vi "PhotogatePiezoMirror.vi"() -> ()   [LabVIEW 2011]
uses:
  <userlib>/atmcd32d.llb/HSSpeed_type typedef.ctl
  <userlib>/atmcd32d.llb/OutputAmplifier_type typedef.ctl
  <vilib>/vision/Image Controls.llb/IMAQ Image.ctl
  <userlib>/atmcd32d.llb/EMGainMode_mode typedef.ctl
  <userlib>/atmcd32d.llb/Shutter_type typedef.ctl
  <userlib>/atmcd32d.llb/Shutter_mode typedef.ctl
  <vilib>/DAQmx/write.llb/DAQmx Write (Analog 1D DBL NChan 1Samp).vi
  <vilib>/DAQmx/write.llb/DAQmx Write (Analog 2D DBL NChan NSamp).vi
  <vilib>/DAQmx/write.llb/DAQmx Write (Digital Bool 1Line 1Point).vi
  <vilib>/DAQmx/create/channels.llb/DAQmx Create Channel (DO-Digital Output).vi
  <vilib>/DAQmx/create/channels.llb/DAQmx Create Channel (AO-Voltage-Basic).vi
  <vilib>/DAQmx/miscellaneous.llb/DAQmx Fill In Error Info.vi
  <vilib>/DAQmx/configure/timing.llb/DAQmx Timing (Sample Clock).vi
  <vilib>/Utility/inputDevices.llb/closeKeyboard.vi
  <vilib>/Utility/inputDevices.llb/keyboardAcquire.vi
  <vilib>/vision/NI_Vision_Development_Module.lvlib
  MCL libraries/MicroDrive.dll
panel:
  in  "Pattern Tab":enum32{"Page 1"}(tab)
  in  "Reset Pattern":bool
  in  "Camera Tab":T1(tab)
  in  "Shutter control":bool=TRUE
  in  "Run pattern":bool
  in  "Control type":T2(ring)
  in  "Mirror pattern params":T3={"Start radius (V)"=1.0, "End radius (V)"=3.0, "Mirror loop rate (Hz)"=200.0, "Ring duration (s)"=1.0, "Ring center X (V)"=0.0, "Ring center Y(V)"=0.0, "Number of spirals"=3, "Time between \ngates (ms)"=0} {"End radius (V)" format="%0.2f"; "Ring center Y(V)" format="%0.2f"; "Ring center X (V)" format="%0.2f"; "Ring duration (s)" format="%0.2f"; "Mirror loop rate (Hz)" format="%0.2f"; "Start radius (V)" format="%0.2f"}
  out "Piezo mirror position":cluster{dbl[], dbl[]}(graph)
  in  "x10":bool
  in  "/10":bool
  in  "Step Size (um)":dbl
  in  "Left":bool
  in  "Right":bool
  in  "Down":bool
  in  "Up":bool
  in  "Zero lower value":bool
  in  "increase jump step size":bool
  in  "decrease jump step size":bool
  in  "Manual Control":bool=TRUE
  in  "Jump step\nsize (um)":dbl=7.0
  in  "Load ROIs":bool
  in  "Standard Pixel Size":bool=TRUE
  out "Main loop running":dbl
  out "Camera starting":dbl
  in  "ROI 128x128":bool
  in  "Reset Scale":bool
  in  "Kill":bool
  out "buffer size":u32 caption="Buf Size"
  in  "Save Note":bool
  in  ".note text control":string
  out "Temp 2":i32 caption="Temp"
  in  "Previous":bool
  in  "Vend":i32=512
  in  "Vstart":i32=1
  in  "Hend":i32=512
  in  "Hstart":i32=1
  in  "Rotate":bool
  in  "Save":bool
  in  "ROI 512x512":bool
  in  "Live":bool
  out "Rate/Hz":u32
  out "# Saved Fr":i32
  out "Act Rate":sgl caption="Calc/Hz"
  out "# images\nin buffer":u32 caption="Buffer / Load"
  out "Buffer":bool
  in  "Auto Scale":bool
  in  "Slide":cluster{dbl, dbl}(slide)={0.0, 5.408163265306123} scale=461.0..773.0
  out "Image 2":T4(plugin-control)
  in  "Image":bool=TRUE
  out "Updating\nImage":bool
  in  "Start Camera":bool
  in  "Pixel Size (nm)":dbl=107.0 caption="pixel"
  in  "Stop Program":bool
  in  "Close Camera":bool
  in  "Direction to move":dbl(knob)
  in  "Time before pattern starts":u32=2000
  out "Current File":string
  in  "File Name":string="stest"
  in  "Folder":path=path "F:/Vlad/122214"
  in  "Gamepad Option":bool
  in  "Save ROIs":bool
  in  "Move with ROI Line":bool
  in  "Base Multiplication Factor":i32=1
  out "Current Speed Multiplication factor":i32
  in  "Max Speed Multiplication Factor":i32=5
  in  "Velocity (mm/s)":dbl=1.5 format="%.3f"
  in  "base step size (um)":dbl=0.2 format="%.3f"
  out "X-Encoder (mm)":dbl format="%.3f"
  out "Y-Encoder (mm)":dbl format="%.3f"
  in  "Photogate":bool
  in  "Piezo mirror X (V)":dbl(slide)=5.0 scale=0.0..10.0
  in  "Piezo mirror Y (V)":dbl(slide)=5.0 scale=0.0..10.0
  out "Piezo mirror\nloop duration (s)":dbl
  in  "Imaging delay (ms)":sgl
  out "Do Stage Jump":bool
  out "keys pressed":T5(array[ring])
  out "First Key":T6(ring)
  in  "Y Increasing":string(combo)="32"
  in  "Y Decreasing":string(combo)="28"
  in  "X Decreasing":string(combo)="10"
  in  "X Increasing":string(combo)="13"
  out "X Reverse Limit":bool
  out "X Forward Limit":bool
  out "Y Reverse Limit":bool
  out "Y Forward Limit":bool
  in  "Reset Y":bool
  in  "Reset  Both":bool
  in  "Reset X":bool
  in  "Time before stage jump":u32=300
  in  "Convert Files":bool
  in  "Analyze Files":bool
  out "List Analyzed":string[](array[string])
  out "List Not Analyzed":string[](array[string])
  in  "Fan Mode":i32(ring)=2 items=["fan on full", "fan on low", "fan off"]
  out "Actual Expsoure":sgl
  in  "Shutter":u16(ring) items=["Auto", "Open", "Closed"]
  in  "PreAmp":i32(ring)=2 items=["1X", "2.5X", "5.4X"]
  in  "VS Speed":i32(ring)=1 items=["0.3 usec", "0.5 usec", "0.9 usec", "1.7 usec", "3.3 usec"]
  in  "HS Speed":i32(ring)=1 items=["10 MHz", "5 MHz", "3 MHz", "1 MHz"]
  in  "Gain":i32=50
  in  "Exposure(ms)":sgl=100.0 format="%#.2f"
  in  "Temp 3":i32=-80 caption="Temperature"
  out "Camera Closing":bool
  out "Program Closing":bool
  out ".note path":path
  in  "16-bit Display Mapping:Conversion Method":u32(ring)=2 items=["Full Dynamic", "Downshift", "Given Range", "90% Dynamic", "Given Percent Range"]
  out "ref image":T4
  in  "Output Amp":T7
  in  "EMCCD":T8
  out "error out 3":errorcluster
  out "Y #pixels":i32
  out "X #pixels":i32
  out "total #pixels":i32
  in  "Trigger":u32(ring) items=["Internal", "External"]
  out "Camera Initialized":bool
  out "His Hstart":i32=1
  out "His Vstart":i32=1
  out "His Hend":i32=1
  out "His Vend":i32=1
  in  "Keep cooler on":bool
  out "frame rate var":i32
  out "tick var":u32
  out "DLL error code":u32
  out "ref image fake":T4
  out "Temp>0":bool
  in  "Base Path":path=path "F:/Vlad"
  out "Saved ROI":T9
  out "Saving File":bool
  in  "timing source":tag="/Dev1/PFI0"
  # "R      G      B       V"
  # "Notes"
  # "Press Ctrl to create the second ROI"
  # "Camera Settings"
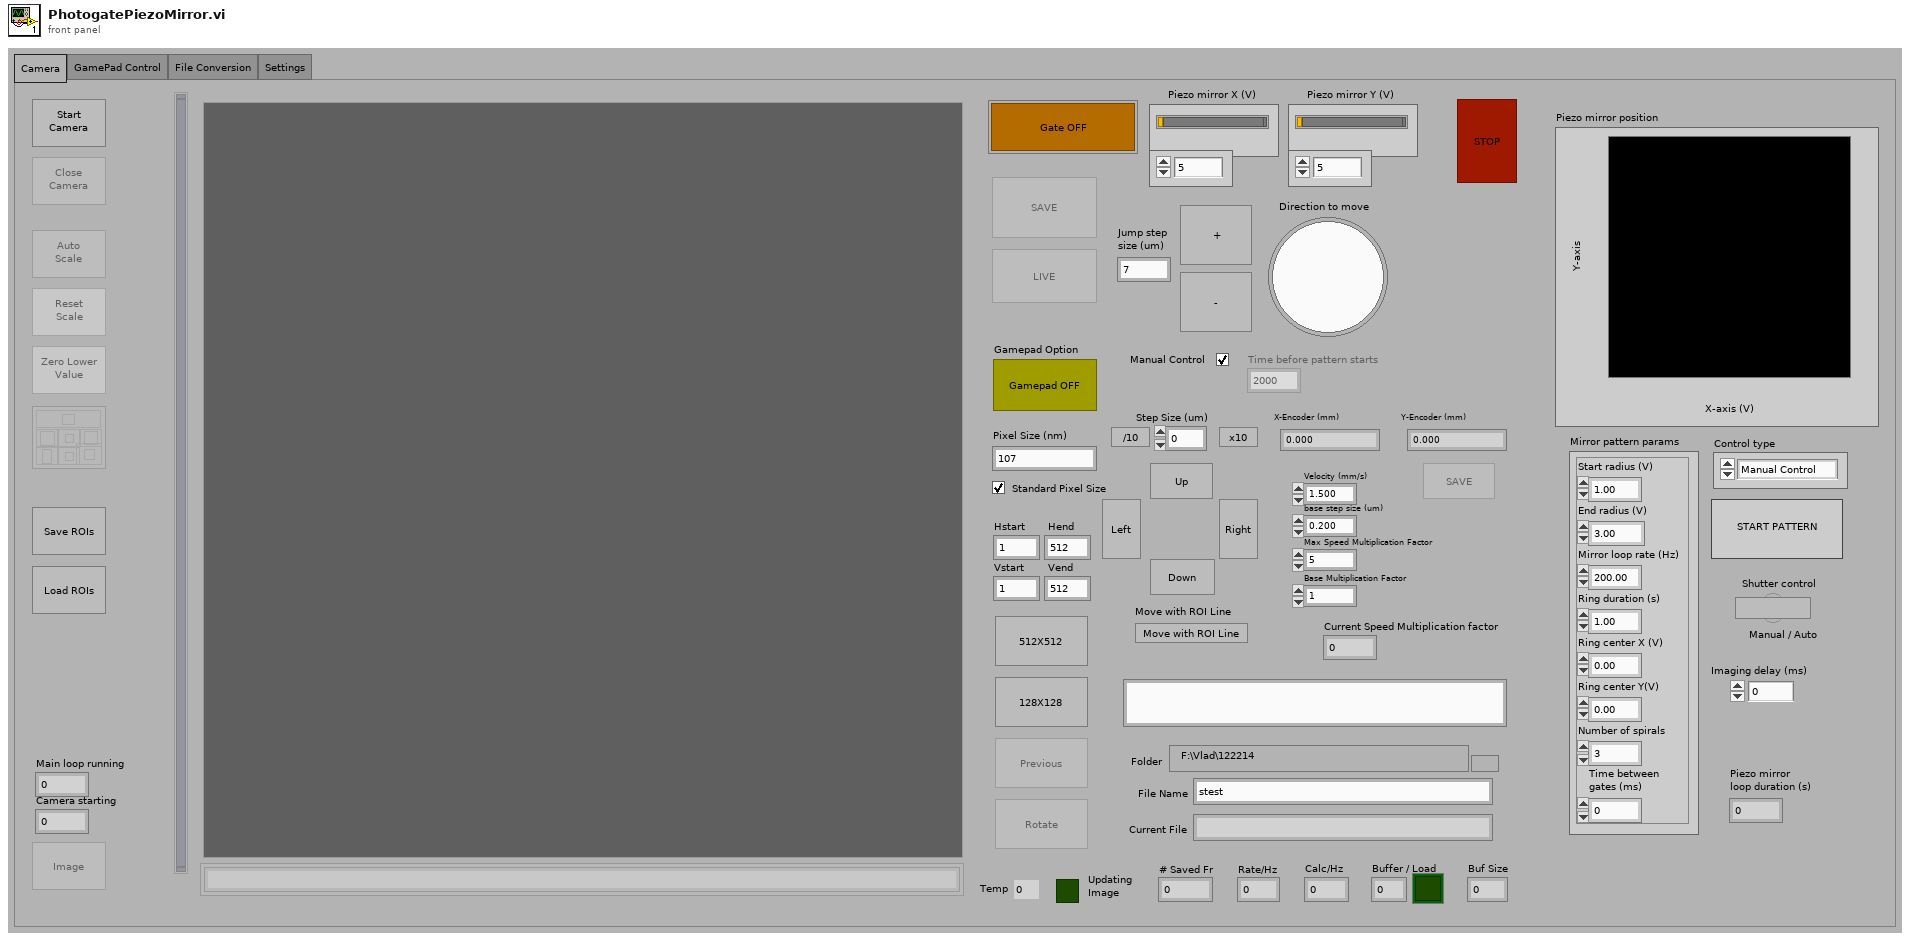
[diagram p1: front panel]
types:
  T1 = enum32{"Camera", "GamePad Control", "File Conversion", "Settings"}
  T2 = enum16{"Manual Control", "Single pattern", "Spiral to circle"}
  T3 = cluster{"Start radius (V)":dbl, "End radius (V)":dbl, "Mirror loop rate (Hz)":dbl, "Ring duration (s)":dbl, "Ring center X (V)":dbl, "Ring center Y(V)":dbl, "Number of spirals":u32, "Time between \ngates (ms)":u32}
  T4 = typedef "IMAQ Image.ctl" = refnum<image>
  T5 = enum16{"0", "1", "2", "3", "4", "5", "6", "7", "8", "9", "A", "B", "C", "D", "E", "F", "G", "H", "I", "J", "K", "L", "M", "N", "O", "P", "Q", "R", "S", "T", "U", "V", "W", "X", "Y", "Z", "F1", "F2", "F3", "F4", "F5", "F6", "F7", "F8", "F9", "F10", "F11", "F12", "F13", "F14", "F15", "ADD", "BACK", "BACKSLASH", "CAPITAL", "COMMA", "DECIMAL", "DELETE", "DIVIDE", "DOWN", "END", "EQUALS", "ESCAPE", "GRAVE (`)", "HOME", "INSERT", "LBRACKET", "LCONTROL", "LEFT", "L ALT", "LSHIFT", "LWIN", "MINUS", "MULTIPLY", "NEXT", "NUMLOCK", "NUMPAD_0", "NUMPAD_1", "NUMPAD_2", "NUMPAD_3", "NUMPAD_4", "NUMPAD_5", "NUMPAD_6", "NUMPAD_7", "NUMPAD_8", "NUMPAD_9", "PAUSE", "PERIOD", "PRIOR (PG UP)", "RBRACKET", "RCONTROL", "RETURN", "RIGHT", "R ALT", "RSHIFT", "RWIN", "SCROLL", "SEMICOLON", "SLASH", "SPACE", "SUBTRACT", "TAB", "UP", "ENTER (num pad)", "' (quote)"}[]
  T6 = enum32{"0", "1", "2", "3", "4", "5", "6", "7", "8", "9", "A", "B", "C", "D", "E", "F", "G", "H", "I", "J", "K", "L", "M", "N", "O", "P", "Q", "R", "S", "T", "U", "V", "W", "X", "Y", "Z", "F1", "F2", "F3", "F4", "F5", "F6", "F7", "F8", "F9", "F10", "F11", "F12", "F13", "F14", "F15", "ADD", "BACK", "BACKSLASH", "CAPITAL", "COMMA", "DECIMAL", "DELETE", "DIVIDE", "DOWN", "END", "EQUALS", "ESCAPE", "GRAVE (`)", "HOME", "INSERT", "LBRACKET", "LCONTROL", "LEFT", "L ALT", "LSHIFT", "LWIN", "MINUS", "MULTIPLY", "NEXT", "NUMLOCK", "NUMPAD_0", "NUMPAD_1", "NUMPAD_2", "NUMPAD_3", "NUMPAD_4", "NUMPAD_5", "NUMPAD_6", "NUMPAD_7", "NUMPAD_8", "NUMPAD_9", "PAUSE", "PERIOD", "PRIOR (PG UP)", "RBRACKET", "RCONTROL", "RETURN", "RIGHT", "R ALT", "RSHIFT", "RWIN", "SCROLL", "SEMICOLON", "SLASH", "SPACE", "SUBTRACT", "TAB", "UP", "ENTER (num pad)", "' (quote)"}
  T7 = typedef "OutputAmplifier_type typedef.ctl" = enum16{"Standard EMCCD gain register", "Conventional CCD register"}
  T8 = typedef "HSSpeed_type typedef.ctl" = enum16{"EM Amp", "Conventional Amp"}
  T9 = cluster{"Global Rectangle":i32[], "Contours":cluster{"Contour Type":u32, "ROI Type":u32, "Points":i32[]}[]}
  T10 = enum8{"Enabled", "Disabled", "Disabled and Grayed Out"}
  T11 = enum16{"open", "replace", "create", "open or create", "replace or create", "replace or create with confirmation"}
  T12 = typedef "Shutter_type typedef.ctl" = enum16{"TTL Low", "TTL High"}
  T13 = typedef "Shutter_mode typedef.ctl" = enum16{"Auto", "Open", "Close"}
  T14 = enum16{"big-endian, network order", "native, host order", "little-endian"}
  T15 = typedef "EMGainMode_mode typedef.ctl" = enum16{"8-bit", "12-bit", "Linear", "Real"}
  T16 = typedef "Image Type" = u32
  T17 = enum16{"0", "1", "2", "3", "4", "5", "6", "7", "8", "9", "A", "B", "C", "D", "E", "F", "G", "H", "I", "J", "K", "L", "M", "N", "O", "P", "Q", "R", "S", "T", "U", "V", "W", "X", "Y", "Z", "F1", "F2", "F3", "F4", "F5", "F6", "F7", "F8", "F9", "F10", "F11", "F12", "F13", "F14", "F15", "ADD", "BACK", "BACKSLASH", "CAPITAL", "COMMA", "DECIMAL", "DELETE", "DIVIDE", "DOWN", "END", "EQUALS", "ESCAPE", "GRAVE (`)", "HOME", "INSERT", "LBRACKET", "LCONTROL", "LEFT", "L ALT", "LSHIFT", "LWIN", "MINUS", "MULTIPLY", "NEXT", "NUMLOCK", "NUMPAD_0", "NUMPAD_1", "NUMPAD_2", "NUMPAD_3", "NUMPAD_4", "NUMPAD_5", "NUMPAD_6", "NUMPAD_7", "NUMPAD_8", "NUMPAD_9", "PAUSE", "PERIOD", "PRIOR (PG UP)", "RBRACKET", "RCONTROL", "RETURN", "RIGHT", "R ALT", "RSHIFT", "RWIN", "SCROLL", "SEMICOLON", "SLASH", "SPACE", "SUBTRACT", "TAB", "UP", "ENTER (num pad)", "' (quote)"}
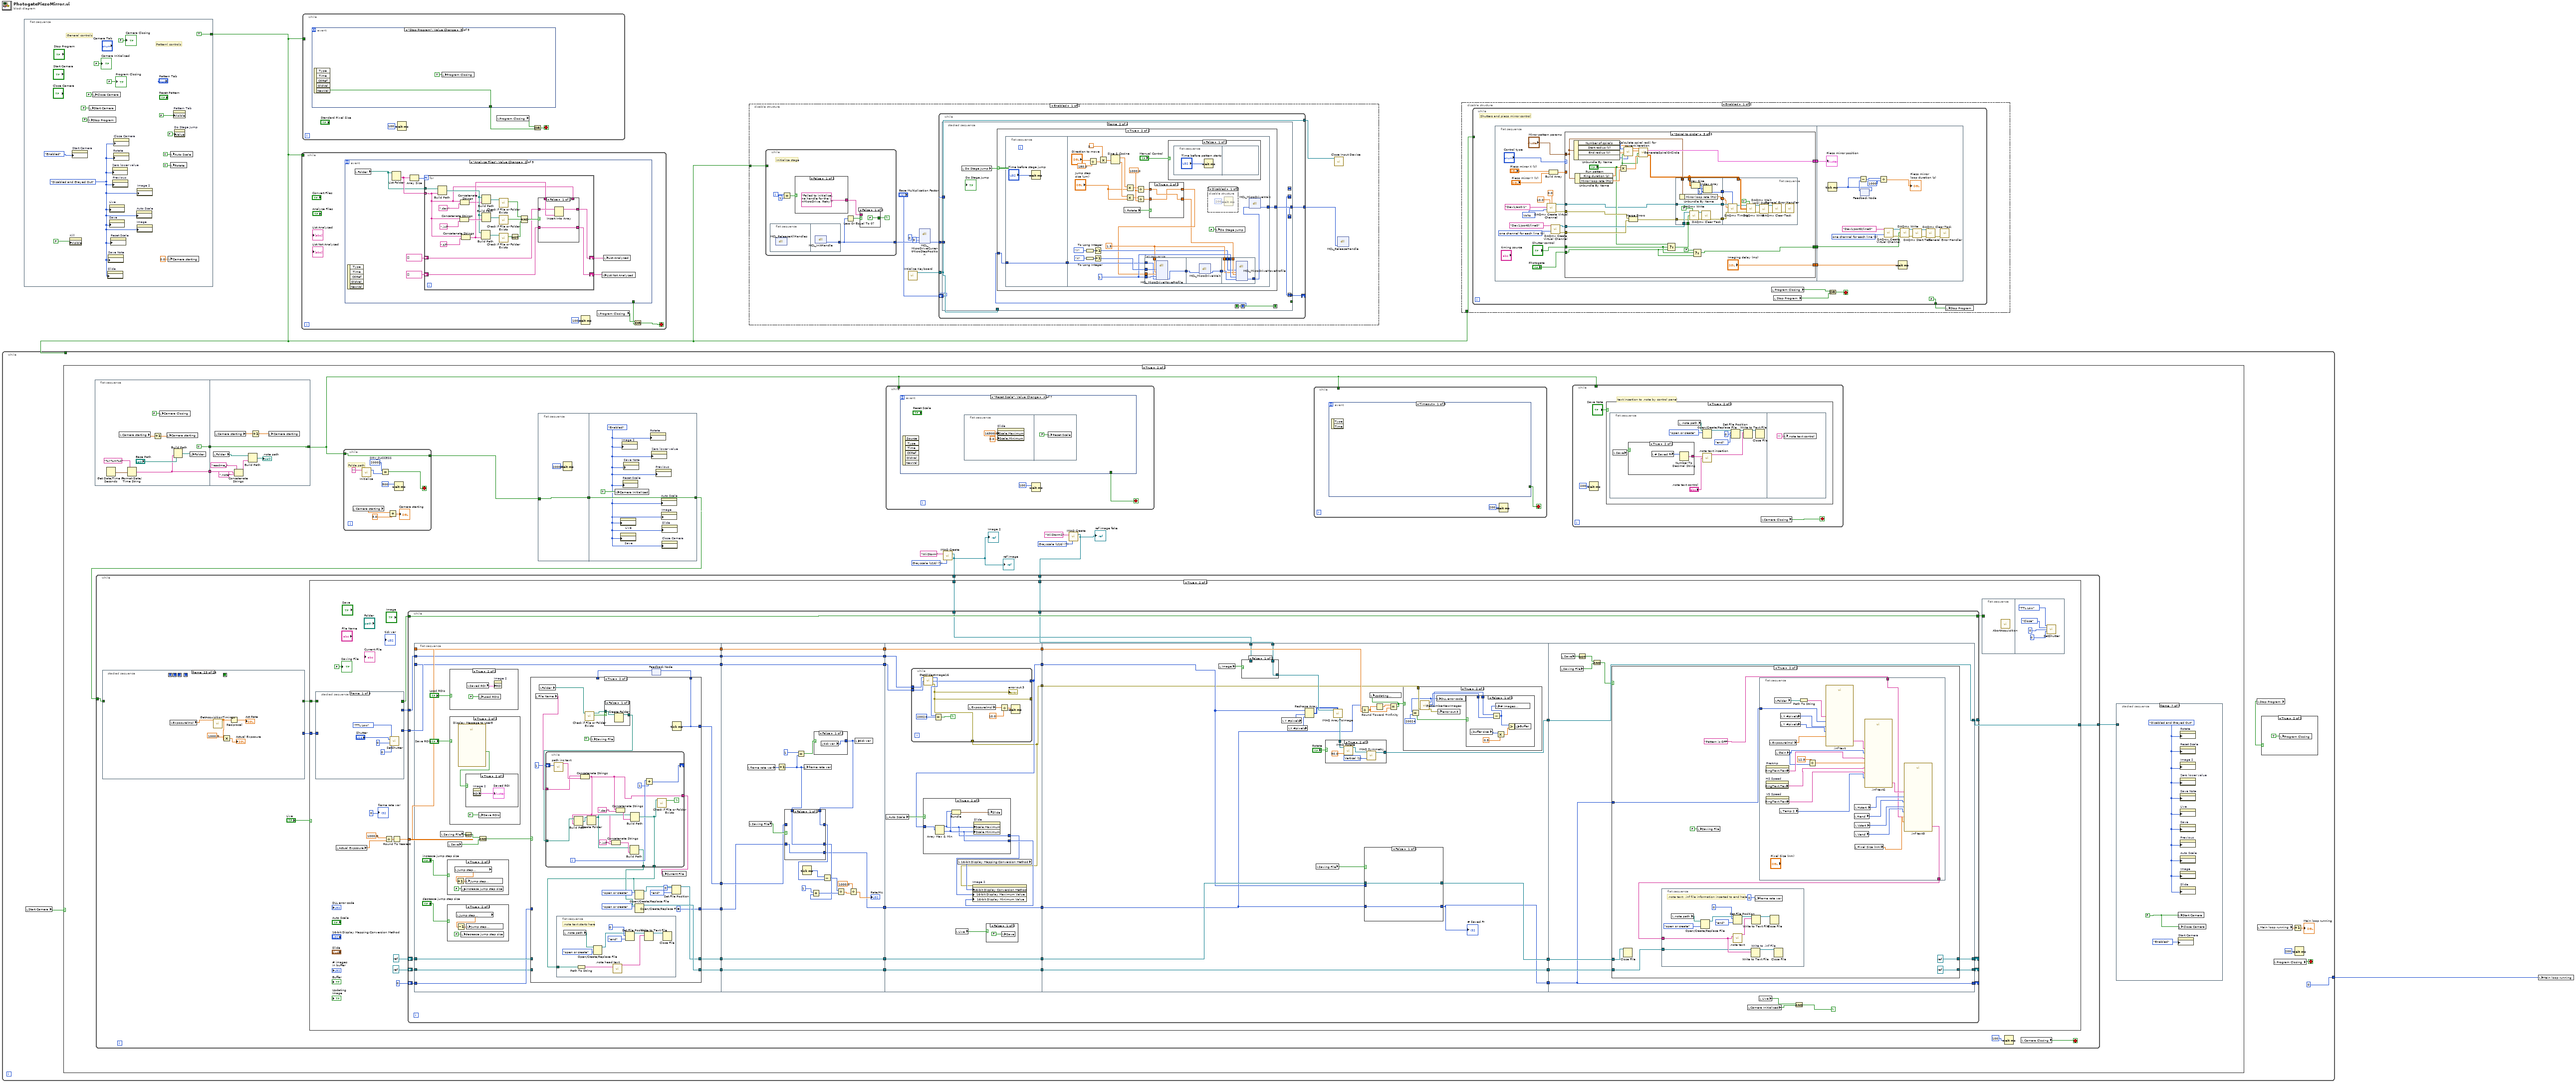
[diagram p0: block diagram]
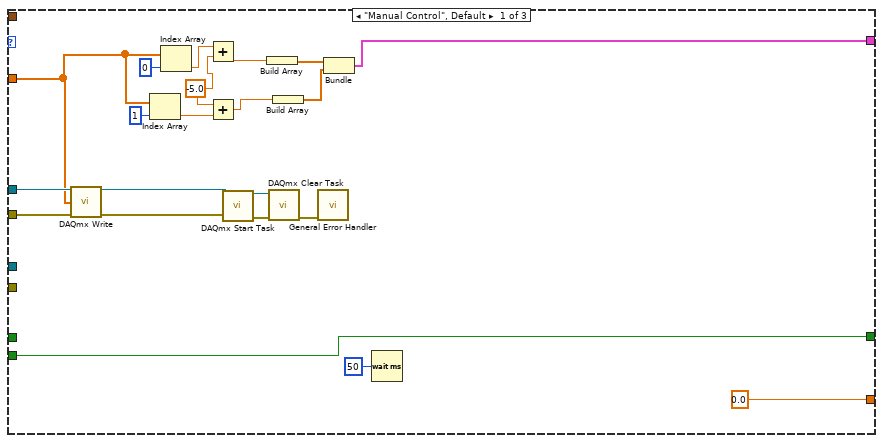
[diagram p2: hidden frame]
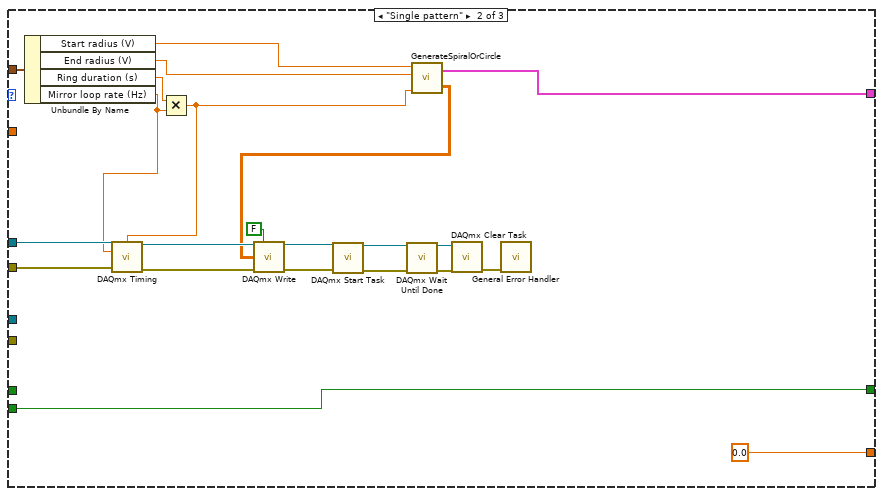
[diagram p3: hidden frame]
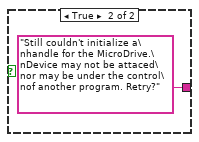
[diagram p5: hidden frame]
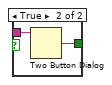
[diagram p6: hidden frame]
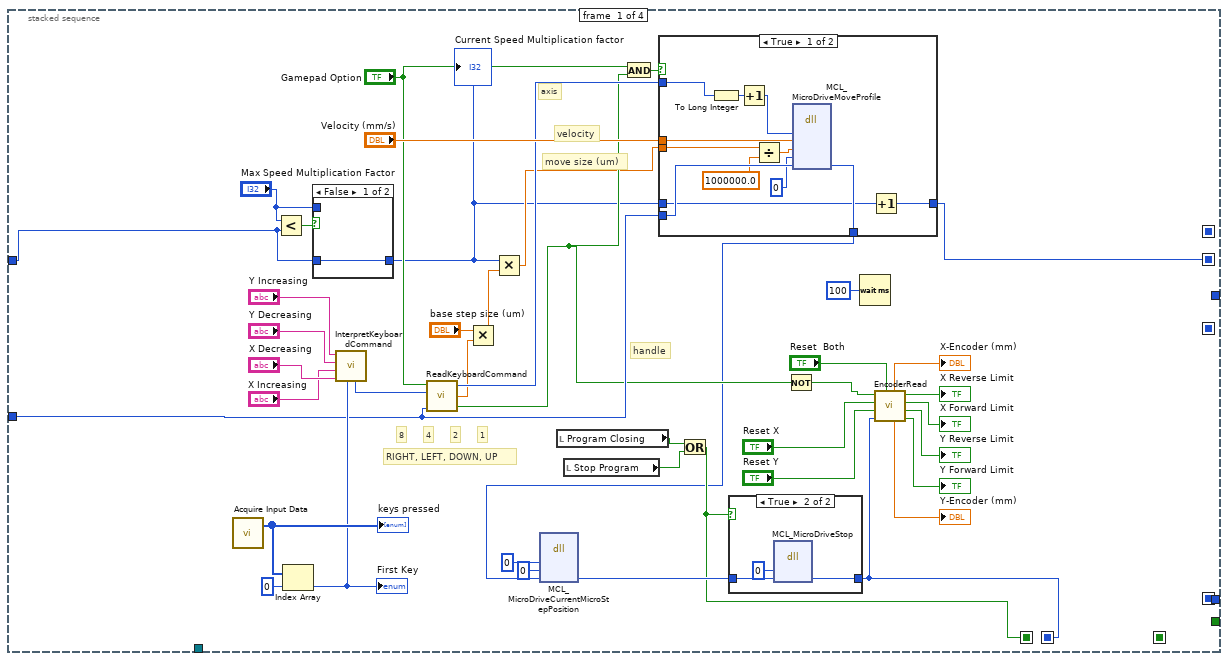
[diagram p7: hidden frame]
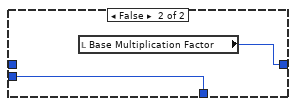
[diagram p9: hidden frame]
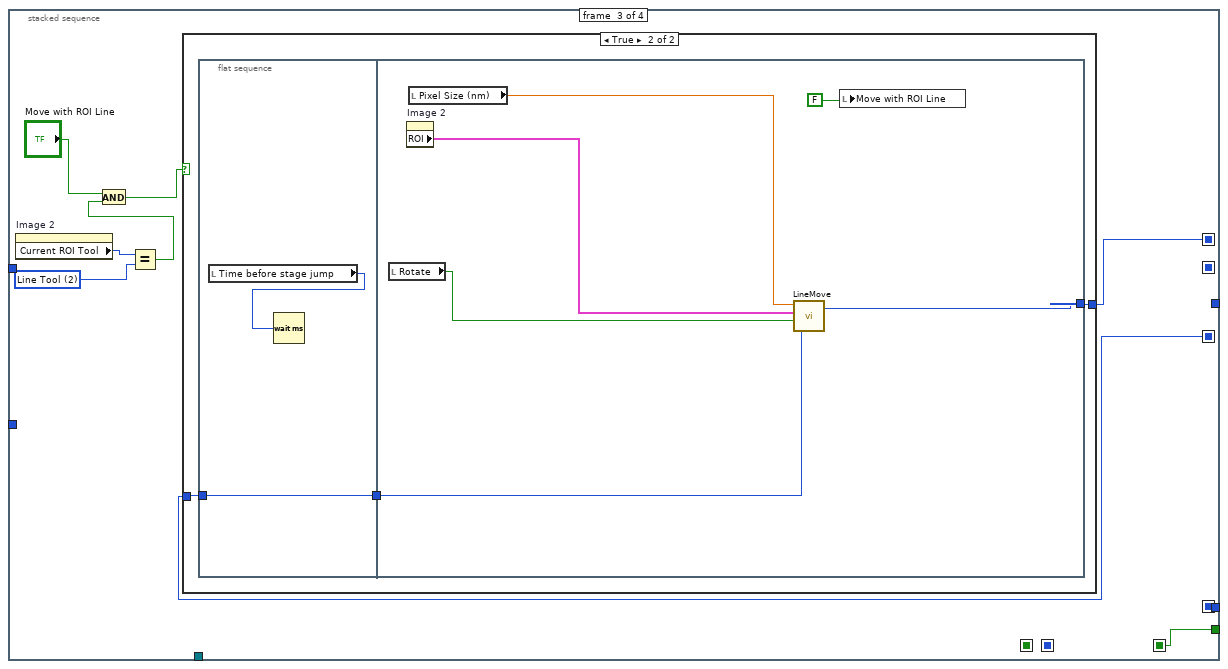
[diagram p15: hidden frame]
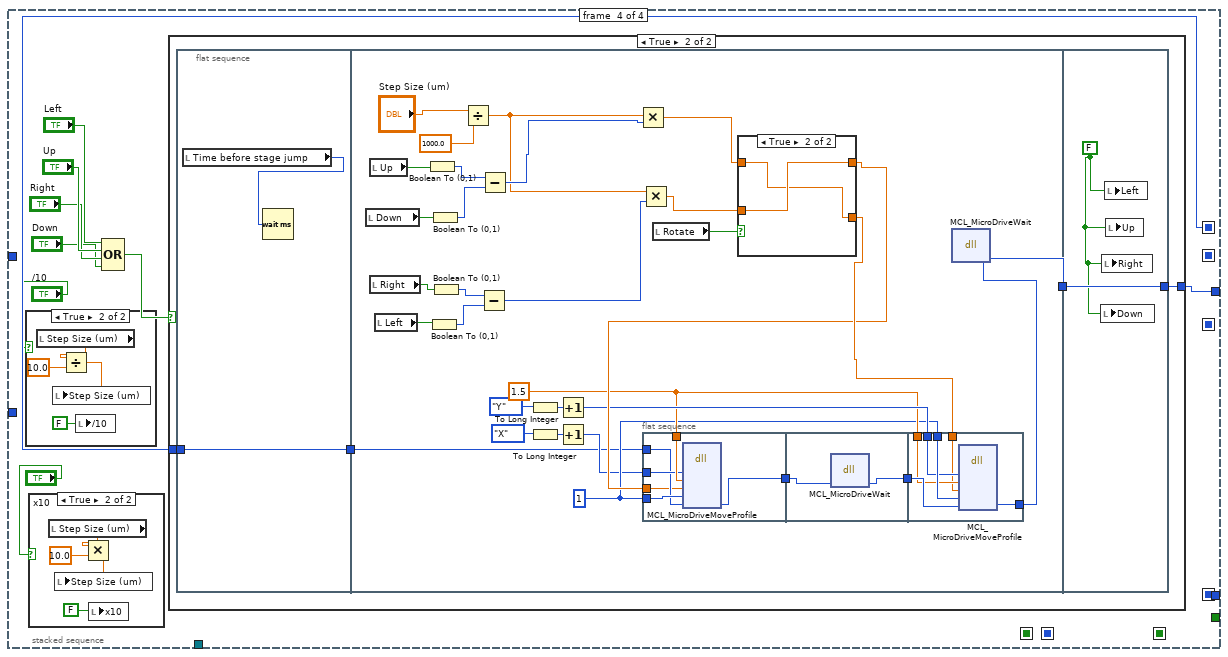
[diagram p17: hidden frame]
diagram:
  n1 = while {
    tunnel: w1 -> [_]
    tunnel: [0] -> w2
    stop <- w7 stop-if-true
    n2 = local read "Start Camera"() -> (w6:bool)
    n3 = case shown="True" w6 {
      frame False {
      }
      frame True {
        w13 = T16 7 items=["Grayscale (U8)", "Grayscale (I16)", "Grayscale (SGL)", "Complex (CSG)", "RGB (U32)", "HSL (U32)", "RGB (U64)", "Grayscale (U16)"] ("Image Type")
        w14 = T16 7 items=["Grayscale (U8)", "Grayscale (I16)", "Grayscale (SGL)", "Complex (CSG)", "RGB (U32)", "HSL (U32)", "RGB (U64)", "Grayscale (U16)"] ("Image Type")
        n4 = flat-sequence {
          tunnel: [TRUE] -> w23
          tunnel: [w97] -> w22
          tunnel: [w110] -> w11
          tunnel: w23 -> [w110]
          tunnel: w22 -> [w107]
          frame #0 {
            n5 = Get Date/Time In Seconds() -> (seconds since 1Jan1904=w100:timestamp)
            n6 = local read "Camera starting"() -> (w95:dbl)
            n7 = Format Date/Time String(time format string (%c)="%Y%m%d", seconds (now)=w100) -> (date/time string=w97:string)  [unwired: 1 in]
            n8 = Increment(x=w95) -> (x+1=w94:dbl)
            n9 = local write "Camera Closing"(FALSE ("Camera Closing")) -> ()
            n10 = local write "Camera starting"(w94) -> ()
            n11 = Build Path(base path="Base Path", name or relative path=w97) -> (appended path=w96:path)
            n12 = local write "Folder"(w96) -> ()
          }
          frame #1 {
            n13 = local read "Folder"() -> (w109:path)
            n14 = local read "Camera starting"() -> (w103:dbl)
            n15 = Concatenate Strings("readme_" ("string"), w107, ".note" ("string")) -> (w108:string)
            n16 = Build Path(base path=w109, name or relative path=w108) -> (appended path=→".note path":path)
            n17 = Increment(x=w103) -> (x+1=w102:dbl)
            n18 = local write "Camera starting"(w102) -> ()
          }
        }
        n19 = while {
          tunnel: [w583] -> w21
          tunnel: w11 -> [w583]
          stop <- w582 stop-if-true
          w585 = 20002  # DRV_SUCCESS
          # "Folde path"
          n20 = local read "Camera starting"() -> (w580:dbl)
          n21 = call <userlib>:"Initialize.vi"("directory (\"\")"="") -> ("DLL error code"=w586:u32)  [unwired: 1 in, 1 out]
          n22 = Equal?(x=w585, y=w586) -> (x = y?=w582:bool)
          n23 = Add(x=w580, y=3.0) -> (x+y=→"Camera starting":dbl)
          n24 = Wait (ms)(milliseconds to wait=u32 500) -> ()  [unwired: 1 out]
        }
        n25 = flat-sequence {
          tunnel: w21 -> [w36]
          tunnel: [w36] -> w12
          tunnel: [w40] -> w20
          tunnel: w12 -> [w40]
          frame #0 {
            n26 = Wait (ms)(milliseconds to wait=u32 2000) -> ()  [unwired: 1 out]
          }
          frame #1 {
            w38 = T10."Enabled" ("Disabled")
            n27 = local write "Camera Initialized"(TRUE ("Camera Initialized")) -> ()
            n28 = property on="Live" class="Bool (strict)"("DisabledEnum"=w38) -> ()  [unwired: 2 in, 2 out]
            n29 = property on="Save" class="Bool (strict)"("DisabledEnum"=w38) -> ()  [unwired: 2 in, 2 out]
            n30 = property on="Image 2" class="ImageControl"("DisabledEnum"=w38) -> ()  [unwired: 2 in, 2 out]
            n31 = property on="Reset Scale" class="Bool (strict)"("DisabledEnum"=w38) -> ()  [unwired: 2 in, 2 out]
            n32 = property on="Save Note" class="Bool"("DisabledEnum"=w38) -> ()  [unwired: 2 in, 2 out]
            n33 = property on="Rotate" class="Bool (strict)"("DisabledEnum"=w38) -> ()  [unwired: 2 in, 2 out]
            n34 = property on="Zero lower value" class="Bool (strict)"("DisabledEnum"=w38) -> ()  [unwired: 2 in, 2 out]
            n35 = property on="Previous" class="Bool"("DisabledEnum"=w38) -> ()  [unwired: 2 in, 2 out]
            n36 = property on="Auto Scale" class="Bool (strict)"("DisabledEnum"=w38) -> ()  [unwired: 2 in, 2 out]
            n37 = property on="Image" class="Bool (strict)"("DisabledEnum"=w38) -> ()  [unwired: 2 in, 2 out]
            n38 = property on="Slide" class="Slide (strict)"("DisabledEnum"=w38) -> ()  [unwired: 2 in, 2 out]
            n39 = property on="Close Camera" class="Bool (strict)"("DisabledEnum"=w38) -> ()  [unwired: 2 in, 2 out]
          }
        }
        n40 = while {
          tunnel: w11 -> [_]
          stop <- w41 stop-if-true
          n41 = event shown="[3] \"Reset Scale\": Value Change" {
            selector: _ -> [_ _ _ _ _ _ _]
            dyn-events: _ -> [_ _ _ _ _ _ _]
            timeout: _ -> [_ _ _ _ _ _ _]
            tunnel: [_ _ _ _ w68 _ w71] -> w41
            event Timeout {
              n42 = event-data() -> ()  [unwired: 1 in, 2 out]
            }
            event "Base Path": Value Change {
              n43 = event-data() -> ()  [unwired: 1 in, 5 out]
              n44 = flat-sequence {
                tunnel: [w46] -> w43
                tunnel: w43 -> [w52]
                frame #0 {
                  n45 = Get Date/Time In Seconds() -> (seconds since 1Jan1904=w48:timestamp)
                  n46 = Format Date/Time String(time format string (%c)="%m%d%y", seconds (now)=w48) -> (date/time string=w46:string)  [unwired: 1 in]
                  n47 = local read "Base Path"() -> (w44:path)
                  n48 = Build Path(base path=w44, name or relative path=w46) -> (appended path=w45:path)
                  n49 = local write "Folder"(w45) -> ()
                }
                frame #1 {
                  n50 = local read "Folder"() -> (w54:path)
                  n51 = Concatenate Strings("readme_" ("string"), w52, ".note" ("string")) -> (w53:string)
                  n52 = Build Path(base path=w54, name or relative path=w53) -> (appended path=w49:path)
                  n53 = local write ".note path"(w49) -> ()
                }
                frame #2 {
                  n54 = call "Display Message to User"() -> ()  [unwired: 10 in, 2 out]
                }
              }
            }
            event "Folder": Value Change {
              n55 = event-data() -> ()  [unwired: 1 in, 5 out]
              n56 = flat-sequence {
                tunnel: [w56] -> w55
                tunnel: w55 -> [w62]
                frame #0 {
                  n57 = Get Date/Time In Seconds() -> (seconds since 1Jan1904=w58:timestamp)
                  n58 = Format Date/Time String(time format string (%c)="%m%d%y", seconds (now)=w58) -> (date/time string=w56:string)  [unwired: 1 in]
                }
                frame #1 {
                  n59 = local read "Folder"() -> (w64:path)
                  n60 = Concatenate Strings("readme_" ("string"), w62, ".note" ("string")) -> (w63:string)
                  n61 = Build Path(base path=w64, name or relative path=w63) -> (appended path=w59:path)
                  n62 = local write ".note path"(w59) -> ()
                }
                frame #2 {
                  n63 = call "Display Message to User2"() -> ()  [unwired: 10 in, 2 out]
                }
              }
            }
            event "Reset Scale": Value Change {
              n64 = event-data() -> ()  [unwired: 1 in, 6 out]
              n65 = flat-sequence {
                frame #0 {
                  n66 = property on="Slide" class="Slide (strict)"("Scale.Maximum"=16500.0 ("Scale.Range:Maximum"), "Scale.Minimum"=0.0 ("Scale.Range:Minimum")) -> ()  [unwired: 2 in, 2 out]
                }
                frame #1 {
                  n67 = local write "Reset Scale"(FALSE ("Reset Scale")) -> ()
                }
              }
            }
            event "Close Camera": Value Change {
              n68 = event-data() -> ("NewVal"=w68:bool)  [unwired: 1 in, 5 out]
            }
            event "Zero lower value": Value Change {
              n69 = event-data() -> ()  [unwired: 1 in, 6 out]
              n70 = flat-sequence {
                frame #0 {
                  n71 = property on="Slide" class="Slide (strict)"("Scale.Minimum"=0.0 ("Scale.Range:Minimum")) -> ()  [unwired: 2 in, 2 out]
                }
                frame #1 {
                  n72 = local write "Zero lower value"(FALSE ("Reset Scale")) -> ()
                }
              }
            }
            event "Stop Program": Value Change {
              n73 = event-data() -> ("NewVal"=w71:bool)  [unwired: 1 in, 5 out]
            }
          }
          n74 = Wait (ms)(milliseconds to wait=u32 100) -> ()  [unwired: 1 out]
        }
        n75 = call "IMAQ Create"("Image Name"="WiiStorm", "Image Type"=w14) -> ("New Image"=w15:T4)  [unwired: 3 in, 1 out]
        "ref image" <- w15
        "Image 2" <- w15
        n76 = call "IMAQ Create"("Image Name"="WiiStorm2", "Image Type"=w13) -> ("New Image"=w16:T4)  [unwired: 3 in, 1 out]
        "ref image fake" <- w16
        n77 = while {
          tunnel: w20 -> [w119]
          tunnel: [w117] -> w19
          tunnel: w15 -> [w113]
          tunnel: w16 -> [w111]
          stop <- w112 stop-if-true
          n78 = stacked-sequence {
            seq-local: [_ _ _ _ _ _ _ _ _ _ _ _ w510 _ _ _ _ _ _ _ _ _ _ _ _ _] -> [_ _ _ _ _ _ _ _ _ _ _ _ _ w530 _ _ _ _ _ _ _ _ _ _ _ _]
            seq-local: [_ _ _ _ _ _ _ _ _ _ _ _ w507 _ _ _ _ _ _ _ _ _ _ _ _ _] -> [_ _ _ _ _ _ _ _ _ _ _ _ _ w529 _ _ _ _ _ _ _ _ _ _ _ _]
            seq-local: [_ _ _ _ _ _ _ _ _ _ _ _ w505 _ _ _ _ _ _ _ _ _ _ _ _ _] -> [_ _ _ _ _ _ _ _ _ _ _ _ _ w528 _ _ _ _ _ _ _ _ _ _ _ _]
            seq-local: [_ _ _ _ _ _ _ _ _ _ _ _ w503 _ _ _ _ _ _ _ _ _ _ _ _ _] -> [_ _ _ _ _ _ _ _ _ _ _ _ _ w527 _ _ _ _ _ _ _ _ _ _ _ _]
            seq-local: [_ _ _ _ _ _ _ _ _ _ _ _ w498 _ _ _ _ _ _ _ _ _ _ _ _ _] -> [_ _ _ _ _ _ _ _ _ _ _ _ _ w526 _ _ _ _ _ _ _ _ _ _ _ _]
            tunnel: w119 -> [_ _ _ _ _ _ _ _ _ _ _ _ _ _ _ _ _ _ _ _ _ w543 _ _ _ _]
            tunnel: [_ _ _ _ _ _ _ _ _ _ _ _ _ _ _ _ _ _ _ _ _ w543 _ _ _ _] -> w118
            tunnel: [_ _ _ _ _ _ _ _ _ _ _ _ w512 _ _ _ _ _ _ _ _ _ _ _ _ _] -> w114
            frame #0 {
              n79 = call <userlib>:"SetTemperature.vi"("temperature"="Temp 3") -> ()  [unwired: 1 in, 2 out]
            }
            frame #1 {
              n80 = call <userlib>:"CoolerON.vi"() -> ()  [unwired: 2 in, 2 out]
            }
            frame #2 {
              n81 = call <userlib>:"SetADChannel.vi"("channel"=0) -> ()  [unwired: 1 in, 2 out]
            }
            frame #3 {
              w456 = u16 7  # AcquisitionMode
              n82 = call <userlib>:"SetAcquisitionMode.vi"("mode"=w456) -> ()  [unwired: 1 in, 2 out]
            }
            frame #4 {
              w457 = u16 4  # ReadMode
              n83 = call <userlib>:"SetReadMode.vi"("mode"=w457) -> ()  [unwired: 1 in, 2 out]
            }
            frame #5 {
              n84 = Divide(x="Exposure(ms)", y=sgl 1000.0) -> (x/y=w459:sgl)
              n85 = call <userlib>:"SetExposureTime.vi"("time"=w459) -> ()  [unwired: 1 in, 2 out]
            }
            frame #6 {
              n86 = call <userlib>:"SetTriggerMode.vi"("mode"="Trigger") -> ()  [unwired: 1 in, 2 out]
            }
            frame #7 {
              n87 = call <userlib>:"SetNumberAccumulations.vi"("number"=1) -> ()  [unwired: 1 in, 2 out]
            }
            frame #8 {
              n88 = call <userlib>:"SetKineticCycleTime.vi"("time"=sgl 0.0) -> ()  [unwired: 1 in, 2 out]
            }
            frame #9 {
              w465 = i32[] [2] items=["No  event", "Click event", "Draw event", "Move event", "Size event", "Scroll event", "Activate event", "Close event", "Double click event"] ("Events list (all)")
              n89 = invoke on="Image 2" class="ImageControl" method="Get Last Event"("Which Events"=w465) -> ("Tool"=w466:i32)  [unwired: 7 in, 7 out]
              n90 = property on="Image 2" class="ImageControl"() -> ("ROI"=w468:T9)  [unwired: 2 in, 2 out]
              n91 = Equal?(x=w466, y=4) -> (x = y?=w464:bool)
              n92 = case shown="True" w464 {
                tunnel: w468 -> [_ w469]
                frame False {
                }
                frame True {
                  n93 = stacked-sequence {
                    tunnel: w469 -> [w485 _]
                    frame #0 {
                      n94 = Unbundle By Name(w485) -> ("Global Rectangle"=w480:i32[])
                      n95 = local read "Hstart"() -> (w475:i32)
                      n96 = local read "Vstart"() -> (w472:i32)
                      n97 = Index Array(array=w480, index=0) -> (element=w479:i32)
                      n98 = Index Array(array=w480, index=1) -> (element=w478:i32)
                      n99 = Index Array(array=w480, index=2) -> (element=w477:i32)
                      n100 = Index Array(array=w480, index=3) -> (element=w476:i32)
                      n101 = Add(x=w477, y=w475) -> (x+y=w474:i32)
                      n102 = Add(x=w472, y=w476) -> (x+y=w470:i32)
                      n103 = Add(x=w475, y=w479) -> (x+y=w473:i32)
                      n104 = Add(x=w472, y=w478) -> (x+y=w471:i32)
                      n105 = local write "Hstart"(w473) -> ()
                      n106 = local write "Vstart"(w471) -> ()
                      n107 = local write "Hend"(w474) -> ()
                      n108 = local write "Vend"(w470) -> ()
                    }
                    frame #1 {
                      w486 = u32 0 items=["Zoom Tool"=8, "Selection Tool"=0, "Pan Tool"=9, "Point Tool"=1, "Line Tool"=2, "Rectangle Tool"=3, "Rotated Rectangle Tool"=12, "Polyline Tool"=10, "Polygon Tool"=5, "Freehand Tool"=11, "Closed Freehand Tool"=6, "Ellipse Tool"=4, "Annulus Tool"=7] ("Current ROI Tool")
                      n109 = property on="Image 2" class="ImageControl"("Rectangle Tool Button Visibile"=FALSE ("ROI Tool Buttons Visibile:Rectangle Tool Button Visibile")) -> ()  [unwired: 2 in, 2 out]
                      n110 = property on="Image 2" class="ImageControl"("Current ROI Tool"=w486) -> ()  [unwired: 2 in, 2 out]
                    }
                  }
                }
              }
            }
            frame #10 {
              n111 = case shown="True" "ROI 512x512" {
                frame False {
                }
                frame True {
                  n112 = local write "Hstart"(1 ("hstart")) -> ()
                  n113 = local write "Vstart"(1 ("hstart")) -> ()
                  n114 = local write "Hend"(512 ("hstart")) -> ()
                  n115 = local write "Vend"(512 ("hstart")) -> ()
                }
              }
            }
            frame #11 {
              n116 = case shown="True" "ROI 128x128" {
                frame False {
                }
                frame True {
                  n117 = local write "Hstart"(1 ("hstart")) -> ()
                  n118 = local write "Vstart"(1 ("hstart")) -> ()
                  n119 = local write "Hend"(128 ("hstart")) -> ()
                  n120 = local write "Vend"(128 ("hstart")) -> ()
                }
              }
            }
            frame #12 {
              w517 = 1 ("hbin")
              n121 = case shown="False" "Previous" {
                tunnel: ["Hstart" w522] -> w509
                tunnel: ["Vend" w525] -> w502
                tunnel: ["Vstart" w524] -> w504
                tunnel: ["Hend" w523] -> w506
                frame False {
                }
                frame True {
                  n122 = local read "His Hstart"() -> (w522:i32)
                  n123 = local read "His Hend"() -> (w523:i32)
                  n124 = local read "His Vstart"() -> (w524:i32)
                  n125 = local read "His Vend"() -> (w525:i32)
                  n126 = local write "Hstart"(w522) -> ()
                  n127 = local write "Vstart"(w524) -> ()
                  n128 = local write "Hend"(w523) -> ()
                  n129 = local write "Vend"(w525) -> ()
                }
              }
              n130 = feedback-in #1(w509) -> ()
              n131 = feedback #1() -> (w510:i32)  [unwired: 1 in]
              n132 = feedback-in #2(w506) -> ()
              n133 = feedback #2() -> (w507:i32)  [unwired: 1 in]
              n134 = feedback-in #3(w504) -> ()
              n135 = feedback #3() -> (w505:i32)  [unwired: 1 in]
              n136 = feedback-in #4(w502) -> ()
              n137 = feedback #4() -> (w503:i32)  [unwired: 1 in]
              n138 = Not Equal?(x=w509, y=w510) -> (x != y?=w508:bool)
              n139 = Not Equal?(x=w506, y=w507) -> (x != y?=w501:bool)
              n140 = Not Equal?(x=w504, y=w505) -> (x != y?=w500:bool)
              n141 = Not Equal?(x=w502, y=w503) -> (x != y?=w499:bool)
              n142 = Subtract(x=w506, y=w509) -> (x-y=w516:i32)
              n143 = Subtract(x=w502, y=w504) -> (x-y=w515:i32)
              n144 = Compound Arithmetic op=OR(w508, w501, w500, w499) -> (w498:bool)
              n145 = Increment(x=w516) -> (x+1=w513:i32)
              "X #pixels" <- w513
              n146 = Increment(x=w515) -> (x+1=w514:i32)
              "Y #pixels" <- w514
              n147 = Multiply(x=w513, y=w514) -> (x*y=w512:i32)
              "total #pixels" <- w512
              n148 = call <userlib>:"SetImage.vi"("hbin"=w517, "vbin"=w517, "hstart"=w509, "hend"=w506, "vstart"=w504, "vend"=w502) -> ()  [unwired: 20 in, 2 out]
            }
            frame #13 {
              n149 = case shown="True" w526 {
                tunnel: w530 -> [_ w534]
                tunnel: w529 -> [_ w533]
                tunnel: w528 -> [_ w532]
                tunnel: w527 -> [_ w531]
                frame False {
                }
                frame True {
                  "His Hstart" <- w534
                  "His Vstart" <- w532
                  "His Hend" <- w533
                  "His Vend" <- w531
                }
              }
            }
            frame #14 {
              n150 = invoke on="Image 2" class="ImageControl" method="Clear ROI"() -> ()  [unwired: 3 in, 3 out]
            }
            frame #15 {
              n151 = call <userlib>:"SetHSSpeed.vi"("index"="HS Speed", "type"="EMCCD") -> ()  [unwired: 2 in, 2 out]
            }
            frame #16 {
              n152 = call <userlib>:"SetVSSpeed.vi"("index"="VS Speed") -> ()  [unwired: 1 in, 2 out]
            }
            frame #17 {
              n153 = call <userlib>:"SetOutputAmplifier.vi"("type"="Output Amp") -> ()  [unwired: 1 in, 2 out]
            }
            frame #18 {
              n154 = call <userlib>:"SetPreAmpGain.vi"("index"="PreAmp") -> ()  [unwired: 1 in, 2 out]
            }
            frame #19 {
              n155 = call <userlib>:"SetFrameTransferMode.vi"("mode"=enum16{"OFF", "ON"}."ON") -> ()  [unwired: 1 in, 2 out]
            }
            frame #20 {
              n156 = call <userlib>:"SetEMGainMode.vi"("mode"=EMGainMode_mode_typedef."Real") -> ()  [unwired: 1 in, 2 out]
            }
            frame #21 {
              n157 = call <userlib>:"SetEMCCDGain.vi"("gain"="Gain") -> ()  [unwired: 1 in, 2 out]
            }
            frame #22 {
              n158 = local read "Exposure(ms)"() -> (w545:sgl)
              n159 = call <userlib>:"GetAcquisitionTimings.vi"("exposure input"=w545) -> ("exposure"=w548:sgl)  [unwired: 10 in, 4 out]
              n160 = Multiply(x=sgl 1000.0, y=w548) -> (x*y=→"Actual Expsoure":sgl)
              n161 = Reciprocal(x=w548) -> (1/x=→"Act Rate":sgl)
            }
            frame #23 {
              n162 = call <userlib>:"GetSizeOfCircularBuffer.vi"() -> ("index"=→"buffer size":u32)  [unwired: 3 in, 2 out]
            }
            frame #24 {
              n163 = call <userlib>:"GetTemperature.vi"() -> ("temperature"=→"Temp 2":i32)  [unwired: 4 in, 3 out]
            }
            frame #25 {
              n164 = call <userlib>:"SetFanMode.vi"("mode"="Fan Mode") -> ()  [unwired: 1 in, 2 out]
            }
          }
          n165 = case shown="True" "Live" {
            tunnel: w118 -> [_ w133]
            tunnel: [w120 w138] -> w117
            tunnel: w114 -> [_ w132]
            tunnel: w113 -> [_ w131]
            tunnel: w111 -> [_ w126]
            frame False {
              n166 = local read "ref image"() -> (w120:T4)
            }
            frame True {
              n167 = stacked-sequence {
                tunnel: [_ _ w451 _] -> w136
                tunnel: [_ _ w449 _] -> w135
                tunnel: [_ _ w450 _] -> w134
                tunnel: w133 -> [_ _ w450 _]
                tunnel: w132 -> [_ _ w449 _]
                frame #0 {
                  n168 = call <userlib>:"SetShutter.vi"("type"=Shutter_type_typedef."TTL Low", "mode"="Shutter", "closingtime"=0, "openingtime"=0) -> ()  [unwired: 10 in, 2 out]
                }
                frame #1 {
                  # "zoom factor"
                  n169 = local read "X #pixels"() -> (w442:i32)
                  n170 = local read "Y #pixels"() -> (w443:i32)
                  n171 = property on="Image 2" class="ImageControl"() -> ("Image Area Height"=w444:u32, "Image Area Width"=w445:u32)  [unwired: 2 in, 2 out]
                  n172 = Max & Min(x=w442, y=w443) -> (max(x,y)=w446:i32)  [unwired: 1 out]
                  n173 = Max & Min(x=w444, y=w445) -> (min(x,y)=w447:u32)  [unwired: 1 out]
                  n174 = Divide(x=w447, y=w446) -> (x/y=w448:dbl)
                  n175 = property on="Image 2" class="ImageControl"("X Zoom"=w448, "Y Zoom"=w448) -> ()  [unwired: 2 in, 2 out]
                }
                frame #2 {
                  n176 = call <userlib>:"StartAcquisition.vi"() -> ()  [unwired: 2 in, 2 out]
                  n177 = Initialize Array(u16 0 ("element"), w449) -> (w451:u16[])
                }
                frame #3 {
                  n178 = property on="Image 2" class="ImageControl"("Rectangle Tool Button Visibile"=TRUE ("ROI Tool Buttons Visibile:Rectangle Tool Button Visibile")) -> ()  [unwired: 2 in, 2 out]
                }
              }
              n179 = local read "Actual Expsoure"() -> (w121:sgl)
              n180 = Divide(x=sgl 1000.0, y=w121) -> (x/y=w128:sgl)
              n181 = Round To Nearest(number=w128) -> (nearest integer value=w127:sgl)
              n182 = while {
                tunnel: w134 -> [w180]
                tunnel: [w181] -> w138
                tunnel: [w180] -> w137
                tunnel: w131 -> [w179]
                tunnel: w136 -> [w178]
                tunnel: w135 -> [w177]
                tunnel: w127 -> [w176]
                tunnel: w126 -> [w175]
                shift-right: [w159] -> _
                shift-left: refnum<file> refnum ("refnum out") -> [w161]
                shift-right: [w158] -> _
                shift-left: refnum<file> refnum ("refnum out") -> [w157]
                shift-right: [w171] -> _
                shift-left: 0 ("frame rate var") -> [w160]
                stop <- w174 continue-if-true
                n183 = flat-sequence {
                  tunnel: w160 -> [w189]
                  tunnel: w176 -> [w199]
                  tunnel: w161 -> [w190]
                  tunnel: w177 -> [w200]
                  tunnel: w178 -> [w201]
                  tunnel: [w201] -> w167
                  tunnel: [w200] -> w166
                  tunnel: [w191] -> w165
                  tunnel: [w192] -> w164
                  tunnel: [w199] -> w163
                  tunnel: [w193] -> w162
                  tunnel: w157 -> [w186]
                  tunnel: [w185] -> w156
                  tunnel: [w281] -> w154
                  tunnel: [w280] -> w153
                  tunnel: [w279] -> w151
                  tunnel: [w266] -> w149
                  tunnel: [w278] -> w147
                  tunnel: w167 -> [w281]
                  tunnel: w166 -> [w280]
                  tunnel: w165 -> [w279]
                  tunnel: w164 -> [w272]
                  tunnel: w163 -> [w278]
                  tunnel: w162 -> [w270]
                  tunnel: w156 -> [w274]
                  tunnel: [w274] -> w145
                  tunnel: w154 -> [w303]
                  tunnel: w153 -> [w302]
                  tunnel: [w301] -> w152
                  tunnel: w151 -> [w308]
                  tunnel: [w308] -> w150
                  tunnel: w149 -> [w307]
                  tunnel: [w307] -> w148
                  tunnel: w147 -> [w306]
                  tunnel: [w306] -> w146
                  tunnel: w145 -> [w305]
                  tunnel: [w305] -> w144
                  tunnel: [w296] -> w143
                  tunnel: w152 -> [w330]
                  tunnel: w150 -> [w349]
                  tunnel: w148 -> [w332]
                  tunnel: w146 -> [w346]
                  tunnel: w179 -> [w337]
                  tunnel: w175 -> [w336]
                  tunnel: [w350] -> w170
                  tunnel: [w348] -> w169
                  tunnel: [w331] -> w168
                  tunnel: w144 -> [w334]
                  tunnel: [w334] -> w155
                  tunnel: w143 -> [w329]
                  tunnel: [w384] -> w171
                  tunnel: [w393] -> w181
                  tunnel: w170 -> [w392]
                  tunnel: w169 -> [w393]
                  tunnel: w168 -> [w384]
                  tunnel: [w387] -> w159
                  tunnel: [w386] -> w158
                  tunnel: w155 -> [w385]
                  frame #0 {
                    n184 = local read "Saving File"() -> (w197:bool)
                    n185 = case shown="True" "increase jump step size" {
                      frame False {
                      }
                      frame True {
                        n186 = local read "Jump step\nsize (um)"() -> (w203:dbl)
                        n187 = Increment(x=w203) -> (x+1=w202:dbl)
                        n188 = local write "increase jump step size"(FALSE ("increase jump step size")) -> ()
                        n189 = local write "Jump step\nsize (um)"(w202) -> ()
                      }
                    }
                    n190 = case shown="True" "decrease jump step size" {
                      frame False {
                      }
                      frame True {
                        n191 = local read "Jump step\nsize (um)"() -> (w206:dbl)
                        n192 = Decrement(x=w206) -> (x-1=w205:dbl)
                        n193 = local write "decrease jump step size"(FALSE ("decrease jump step size")) -> ()
                        n194 = local write "Jump step\nsize (um)"(w205) -> ()
                      }
                    }
                    n195 = local read "Save"() -> (w195:bool)
                    n196 = case shown="True" "Load ROIs" {
                      frame False {
                      }
                      frame True {
                        n197 = local read "Saved ROI"() -> (w211:T9)
                        n198 = local write "Load ROIs"(FALSE ("Set Ref. Circles")) -> ()
                        n199 = property on="Image 2" class="ImageControl"("ROI"=w211) -> ()  [unwired: 2 in, 2 out]
                      }
                    }
                    n200 = case shown="True" "Save ROIs" {
                      frame False {
                      }
                      frame True {
                        n201 = call "Display Message to User3"() -> ("Yes"=w208:bool)  [unwired: 10 in, 1 out]
                        n202 = case shown="True" w208 {
                          frame False {
                          }
                          frame True {
                            n203 = property on="Image 2" class="ImageControl"() -> ("ROI"=→"Saved ROI":T9)  [unwired: 2 in, 2 out]
                          }
                        }
                        n204 = local write "Save ROIs"(FALSE ("Set Ref. Circles")) -> ()
                      }
                    }
                    n205 = Not(x=w197) -> (.not. x?=w196:bool)
                    n206 = And(x=w196, y=w195) -> (x .and. y?=w194:bool)
                    n207 = feedback #5() -> (w184:u32)  [unwired: 1 in]
                    n208 = case shown="True" w194 {
                      tunnel: [w215 w233] -> w185
                      tunnel: [w216 w229] -> w191
                      tunnel: w190 -> [w216 _]
                      tunnel: w186 -> [w215 _]
                      tunnel: w189 -> [w214 _]
                      tunnel: [w214 0 ("frame rate var")] -> w193
                      tunnel: [w213 w227] -> w198
                      tunnel: w184 -> [w213 _]
                      tunnel: [w213 w227] -> w192
                      frame False {
                      }
                      frame True {
                        n209 = local read "File Name"() -> (w223:string)
                        n210 = local read "Folder"() -> (w222:path)
                        n211 = flat-sequence {
                          tunnel: w219 -> [w256]
                          frame #0 {
                            # ".note text starts here"
                            n212 = local read ".note path"() -> (w262:path)
                            n213 = Path To String(path=w256) -> (string=w257:string)
                            n214 = Open/Create/Replace File(file path (use dialog)=w262, operation (0:open)=T11."open or create") -> (refnum out=w261:refnum<file>)  [unwired: 4 in, 2 out]
                            n215 = call ".note head text"(".daxfilepath"=w257) -> ("Result"=w258:string)  [unwired: 13 in, 1 out]
                            n216 = Set File Position(offset (in bytes) (0)=i64 0, refnum=w261, from (0:start)=enum16{"start", "end", "current"}."end") -> (refnum out=w260:refnum<file>)  [unwired: 1 in, 1 out]
                            n217 = Write to Text File(file (use dialog)=w260, text=w258) -> (refnum out=w259:refnum<file>)  [unwired: 2 in, 2 out]
                            n218 = Close File(refnum=w259) -> ()  [unwired: 1 in, 2 out]
                          }
                        }
                        n219 = call <vilib>:"Check if File or Folder Exists.vi"("path"=w222) -> ("file or folder exists?"=w225:bool, "dup path"=w226:path)  [unwired: 8 in, 1 out]
                        n220 = local write "Saving File"(TRUE ("Saving File")) -> ()
                        n221 = case shown="False" w225 {
                          tunnel: [w237 w238] -> w224
                          tunnel: w226 -> [w236 w238]
                          frame False {
                            n222 = Create Folder(path (use dialog)=w236) -> (created path=w237:path)  [unwired: 2 in, 2 out]
                          }
                          frame True {
                          }
                        }
                        n223 = while {
                          tunnel: [w254] -> w219
                          shift-right: [w249] -> _
                          shift-left: 1 -> [w255]
                          tunnel: w224 -> [w243]
                          tunnel: [w244] -> w221
                          tunnel: w223 -> [w240]
                          tunnel: [w239] -> w220
                          i -> [w251]
                          stop <- w253 continue-if-true
                          n224 = call "path inc text"("inc"=w255) -> ("Result"=w252:string)  [unwired: 13 in, 1 out]
                          n225 = Concatenate Strings(w240, w252) -> (w239:string)
                          n226 = Build Path(base path=w243, name or relative path=w239) -> (appended path=w242:path)
                          n227 = Create Folder(path (use dialog)=w242) -> (created path=w241:path)  [unwired: 2 in, 2 out]
                          n228 = Concatenate Strings(w239, ".inf" ("string")) -> (w245:string)
                          n229 = Concatenate Strings(w239, ".dax" ("string")) -> (w247:string)
                          n230 = Build Path(base path=w241, name or relative path=w245) -> (appended path=w244:path)
                          n231 = Build Path(base path=w241, name or relative path=w247) -> (appended path=w254:path)
                          n232 = Add(x=w251, y=1) -> (x+y=w249:i32)
                          n233 = call <vilib>:"Check if File or Folder Exists.vi"("path"=w254) -> ("file or folder exists?"=w253:bool)  [unwired: 8 in, 2 out]
                        }
                        n234 = Open/Create/Replace File(file path (use dialog)=w219, operation (0:open)=T11."open or create") -> (refnum out=w231:refnum<file>)  [unwired: 4 in, 2 out]
                        n235 = Open/Create/Replace File(file path (use dialog)=w221, operation (0:open)=T11."open or create") -> (refnum out=w233:refnum<file>)  [unwired: 4 in, 2 out]
                        n236 = local write "Current File"(w220) -> ()
                        n237 = Set File Position(offset (in bytes) (0)=i64 0, refnum=w231, from (0:start)=enum16{"start", "end", "current"}."end") -> (refnum out=w229:refnum<file>)  [unwired: 1 in, 1 out]
                        n238 = Tick Count (ms)() -> (millisecond timer value=w227:u32)
                      }
                    }
                    n239 = feedback-in #5(w198) -> ()
                  }
                  frame #1 {
                    n240 = local read "frame rate var"() -> (w277:i32)
                    n241 = local read "Saving File"() -> (w273:bool)
                    n242 = Increment(x=w277) -> (x+1=w267:i32)
                    n243 = Equal?(x=1, y=w267) -> (x = y?=w275:bool)
                    n244 = Tick Count (ms)() -> (millisecond timer value=w282:u32)
                    n245 = local write "frame rate var"(w267) -> ()
                    n246 = case shown="False" w275 {
                      tunnel: [w294 w295] -> w268
                      frame False {
                        n247 = local read "tick var"() -> (w294:u32)
                      }
                      frame True {
                        n248 = Tick Count (ms)() -> (millisecond timer value=w295:u32)
                      }
                    }
                    n249 = case shown="False" w273 {
                      tunnel: w272 -> [_ w293]
                      tunnel: [w291 w293] -> w271
                      tunnel: w270 -> [w289 w292]
                      tunnel: [w290 w292] -> w269
                      tunnel: w268 -> [w291 _]
                      tunnel: w267 -> [w290 _]
                      tunnel: [w289 w292] -> w266
                      frame False {
                      }
                      frame True {
                      }
                    }
                    n250 = Add(x=1, y=w269) -> (x+y=w288:i32)
                    n251 = Subtract(x=w282, y=w271) -> (x-y=w286:u32)
                    n252 = Divide(x=w286, y=w288) -> (x/y=w284:dbl)
                    n253 = Divide(x=1000.0, y=w284) -> (x/y=→"Rate/Hz":dbl)
                    n254 = local write "tick var"(w268) -> ()
                  }
                  frame #2 {
                    n255 = local read "Auto Scale"() -> (w304:bool)
                    n256 = while {
                      tunnel: [w313] -> w301
                      tunnel: w303 -> [w312]
                      tunnel: w302 -> [w314]
                      tunnel: [w311] -> _
                      tunnel: [w311] -> w296
                      stop <- w319 continue-if-true
                      n257 = call <userlib>:"GetOldestImage16.vi"("size"=w314, "array"=w312) -> ("error out"=w311:errorcluster, "array"=w313:u16[], "DLL error code"=w318:u32)  [unwired: 1 in]
                      "error out 3" <- w311
                      n258 = Equal?(x=w318, y=u32 20024) -> (x = y?=w319:bool)
                      n259 = local read "Exposure(ms)"() -> (w310:sgl)
                      n260 = Divide(x=w310, y=sgl 10.0) -> (x/y=w316:sgl)
                      n261 = Wait (ms)(milliseconds to wait=w316) -> ()  [unwired: 1 out]
                    }
                    n262 = case shown="True" w304 {
                      tunnel: w301 -> [_ w328]
                      tunnel: [w321 w325] -> w297
                      tunnel: [w320 w326] -> w298
                      frame False {
                        n263 = local read "Slide"() -> (w324:cluster{dbl, dbl})
                        n264 = Unbundle(w324) -> (w323:dbl, w322:dbl)
                        n265 = To Unsigned Word Integer(number=w323) -> (unsigned 16bit integer=w321:u16)
                        n266 = To Unsigned Word Integer(number=w322) -> (unsigned 16bit integer=w320:u16)
                      }
                      frame True {
                        n267 = Array Max & Min(array=w328) -> (max value=w325:u16, min value=w326:u16)  [unwired: 2 out]
                        n268 = Bundle(w325, w326) -> (w327:cluster{u16, u16})  [unwired: 1 in]
                        n269 = property on="Slide" class="Slide (strict)"("Scale.Maximum"=w325, "Scale.Minimum"=w326) -> ()  [unwired: 2 in, 2 out]
                        n270 = local write "Slide"(w327) -> ()
                      }
                    }
                    n271 = local read "Live"() -> (w300:bool)
                    n272 = local read "16-bit Display Mapping:Conversion Method"() -> (w299:u32)
                    n273 = property on="Image 2" class="ImageControl"(error in=w296, "16-bit Display Conversion Method"=w299, "16-bit Display Maximum Value"=w297, "16-bit Display Minimum Value"=w298) -> ()  [unwired: 1 in, 2 out]
                    n274 = case shown="False" w300 {
                      frame False {
                        n275 = local write "Save"(FALSE) -> ()
                      }
                      frame True {
                      }
                    }
                  }
                  frame #3 {
                    n276 = local read "Image"() -> (w335:bool)
                    n277 = case shown="False" w335 {
                      tunnel: [w382 w383] -> w347
                      tunnel: w337 -> [_ w383]
                      tunnel: w336 -> [w382 _]
                      frame False {
                      }
                      frame True {
                      }
                    }
                    n278 = local read "Y #pixels"() -> (w345:i32)
                    n279 = local read "X #pixels"() -> (w344:i32)
                    n280 = Reshape Array(w330, w345, w344) -> (w339:u16[][])
                    n281 = local read "Saving File"() -> (w333:bool)
                    n282 = call "IMAQ ArrayToImage"("Image Pixels (U16)"=w339, "Image"=w347) -> ("Image Out"=w343:T4)  [unwired: 8 in, 1 out]
                    n283 = case shown="True" "Rotate" {
                      tunnel: w343 -> [w376 w378]
                      tunnel: [w376 w377] -> w348
                      frame False {
                      }
                      frame True {
                        w379 = u32 1 items=["Horizontal", "Vertical", "Central", "1st Diagonal", "2nd Diagonal"] ("Type of Symmetry")
                        n284 = call "IMAQ Rotate"("Angle (degrees)"=sgl 90.0, "Image Src"=w378) -> ("Image Dst Out"=w380:T4)  [unwired: 8 in, 1 out]
                        n285 = call "IMAQ Symmetry"("Type of Symmetry"=w379, "Image Src"=w380) -> ("Image Dst Out"=w377:T4)  [unwired: 3 in, 1 out]
                      }
                    }
                    n286 = Divide(x=w332, y=w346) -> (x/y=w341:sgl)
                    n287 = case shown="False" w333 {
                      tunnel: [w352 w359] -> w350
                      tunnel: w349 -> [w352 w358]
                      tunnel: w330 -> [_ w357]
                      tunnel: w332 -> [w351 w354]
                      tunnel: [w351 w353] -> w331
                      frame False {
                      }
                      frame True {
                        # "save file"
                        n288 = Increment(x=w354) -> (x+1=w353:i32)
                        n289 = Write to Binary File(file (use dialog)=w358, data=w357, 5:FALSE ("prepend array or string size? (T)"), 9:T14."big-endian, network order" ("byte order (0:big-endian, network order)")) -> (refnum out=w359:refnum<file>)  [unwired: 2 in, 2 out]
                      }
                    }
                    "# Saved Fr" <- w331
                    n290 = Round Toward +Infinity(x=w341) -> (ceil(x): smallest int >= x=w342:sgl)
                    n291 = Equal?(x=w342, y=w341) -> (x = y?=w340:bool)
                    n292 = local write "Updating\nImage"(w340) -> ()
                    n293 = case shown="True" w340 {
                      tunnel: w329 -> [_ w364]
                      frame False {
                      }
                      frame True {
                        n294 = call <userlib>:"GetNumberNewImages.vi"("error in (no error)"=w364) -> ("error out"=w363:errorcluster, "last"=w365:i32, "first"=w366:u32, "DLL error code"=w360:u32)  [unwired: 3 in]
                        n295 = Equal?(x=w360, y=u32 20024) -> (x = y?=w361:bool)
                        n296 = local write "DLL error code"(w360) -> ()
                        n297 = local write "error out 3"(w363) -> ()
                        n298 = case shown="False" w361 {
                          tunnel: w366 -> [w373 _]
                          tunnel: w365 -> [w372 _]
                          frame False {
                            n299 = local read "buffer size"() -> (w371:u32)
                            n300 = Subtract(x=w372, y=w373) -> (x-y=w367:u32)
                            n301 = local write "# images\nin buffer"(w367) -> ()
                            n302 = Multiply(x=w371, y=0.5) -> (x*y=w369:dbl)
                            n303 = Greater?(x=w367, y=w369) -> (0:w368:bool)
                            n304 = local write "Buffer"(w368) -> ()
                          }
                          frame True {
                            n305 = local write "# images\nin buffer"(u32 0 ("# images\nin buffer")) -> ()
                            n306 = local write "Buffer"(FALSE ("Buffer")) -> ()
                          }
                        }
                      }
                    }
                  }
                  frame #4 {
                    n307 = local read "Saving File"() -> (w390:bool)
                    n308 = local read "Save"() -> (w389:bool)
                    n309 = Not(x=w389) -> (.not. x?=w391:bool)
                    n310 = And(x=w391, y=w390) -> (x .and. y?=w388:bool)
                    n311 = case shown="True" w388 {
                      tunnel: w384 -> [_ w401]
                      tunnel: w385 -> [w394 w400]
                      tunnel: [w395 refnum<file> refnum ("refnum out")] -> w387
                      tunnel: [w394 refnum<file> refnum ("refnum out")] -> w386
                      tunnel: w392 -> [w395 w399]
                      frame False {
                      }
                      frame True {
                        n312 = Close File(refnum=w399) -> ()  [unwired: 1 in, 2 out]
                        n313 = flat-sequence {
                          tunnel: w402 -> [w428]
                          tunnel: w400 -> [w427]
                          frame #0 {
                            # ".note text: .inf file information inserted to end here"
                            n314 = local read ".note path"() -> (w434:path)
                            n315 = Open/Create/Replace File(file path (use dialog)=w434, operation (0:open)=T11."open or create") -> (refnum out=w433:refnum<file>)  [unwired: 4 in, 2 out]
                            n316 = Set File Position(offset (in bytes) (0)=i64 0, refnum=w433, from (0:start)=enum16{"start", "end", "current"}."end") -> (refnum out=w432:refnum<file>)  [unwired: 1 in, 1 out]
                            n317 = call ".note text"(".inf"=w428) -> ("Result"=w431:string)  [unwired: 13 in, 1 out]
                            n318 = Write to Text File "Write to .inf File"(file (use dialog)=w427, text=w428) -> (refnum out=w429:refnum<file>)  [unwired: 2 in, 2 out]
                            n319 = Write to Text File(file (use dialog)=w432, text=w431) -> (refnum out=w430:refnum<file>)  [unwired: 2 in, 2 out]
                            n320 = local write "frame rate var"(0 ("frame rate var")) -> ()
                            n321 = Close File(refnum=w430) -> ()  [unwired: 1 in, 2 out]
                            n322 = Close File(refnum=w429) -> ()  [unwired: 1 in, 2 out]
                          }
                        }
                        n323 = local write "Saving File"(FALSE ("Saving File")) -> ()
                        n324 = flat-sequence {
                          tunnel: "Pattern is OFF" -> [w410]
                          tunnel: [w409] -> w402
                          tunnel: w401 -> [w422]
                          frame #0 {
                            n325 = property on="HS Speed" class="Ring (strict)"() -> ("RingText.Text"=w405:string)  [unwired: 2 in, 2 out]
                            n326 = property on="PreAmp" class="Ring (strict)"() -> ("RingText.Text"=w407:string)  [unwired: 2 in, 2 out]
                            n327 = property on="VS Speed" class="Ring (strict)"() -> ("RingText.Text"=w404:string)  [unwired: 2 in, 2 out]
                            n328 = local read "Exposure(ms)"() -> (w408:sgl)
                            n329 = local read "Folder"() -> (w424:path)
                            n330 = local read "Gain"() -> (w406:i32)
                            n331 = local read "Temp 2"() -> (w417:i32)
                            n332 = local read "X #pixels"() -> (w421:i32)
                            n333 = local read "Y #pixels"() -> (w420:i32)
                            n334 = Path To String(path=w424) -> (string=w423:string)
                            n335 = Divide(x=12.5, y=w406) -> (x/y=w418:dbl)
                            n336 = call ".inf text"("h"=w420, "path"=w423, "frames"=w422, "w"=w421, "exposure"=w408) -> ("Result"=w419:string)  [unwired: 9 in, 1 out]
                            n337 = local read "Hend"() -> (w414:i32)
                            n338 = local read "Hstart"() -> (w415:i32)
                            n339 = local read "Vstart"() -> (w413:i32)
                            n340 = local read "Vend"() -> (w412:i32)
                            n341 = local read "Pixel Size (nm)"() -> (w411:dbl)
                            n342 = call ".inf text2"("Beginning Text"=w419, "hsspeed"=w405, "temperature"=w417, "gain"=w406, "preampgain"=w407, "photonconversion"=w418, "vsspeed"=w404) -> ("Result"=w416:string)  [unwired: 7 in, 1 out]
                            n343 = call ".inf text3"("Beginning Text"=w416, "vend"=w412, "pixelsize"=w411, "hstart"=w415, "hend"=w414, "vstart"=w413, "pattern"=w410) -> ("Result"=w409:string)  [unwired: 7 in, 1 out]
                          }
                        }
                      }
                    }
                  }
                }
                n344 = local read "Camera Initialized"() -> (w172:bool)
                n345 = local read "Live"() -> (w173:bool)
                n346 = And(x=w173, y=w172) -> (x .and. y?=w174:bool)
              }
              n347 = flat-sequence {
                tunnel: w137 -> [_]
                frame #0 {
                  n348 = call <userlib>:"AbortAcquisition.vi"() -> ()  [unwired: 2 in, 2 out]
                }
                frame #1 {
                  n349 = call <userlib>:"SetShutter.vi"("type"=Shutter_type_typedef."TTL Low", "mode"=Shutter_mode_typedef."Close", "closingtime"=0, "openingtime"=0) -> ()  [unwired: 10 in, 2 out]
                }
              }
              "frame rate var" <- 0 ("frame rate var")
              "Saving File" <- FALSE ("Saving File")
            }
          }
          n350 = Wait (ms)(milliseconds to wait=u32 100) -> ()  [unwired: 1 out]
          n351 = local read "Camera Closing"() -> (w112:bool)
        }
        n352 = while {
          tunnel: w11 -> [_]
          stop <- w25 stop-if-true
          n353 = event shown="[0] Timeout" {
            selector: _ -> [_ _ _]
            dyn-events: _ -> [_ _ _]
            timeout: _ -> [_ _ _]
            tunnel: [_ w26 w28] -> w25
            event Timeout {
              n354 = event-data() -> ()  [unwired: 1 in, 2 out]
            }
            event "Stop Program": Value Change {
              n355 = event-data() -> ("NewVal"=w26:bool)  [unwired: 1 in, 4 out]
              n356 = case shown="True" w26 {
                frame False {
                }
                frame True {
                  n357 = local write "Camera Closing"(TRUE ("Program Closing")) -> ()
                }
              }
            }
            event "Close Camera": Value Change {
              n358 = event-data() -> ("NewVal"=w29:bool)  [unwired: 1 in, 4 out]
              n359 = case shown="True" w29 {
                tunnel: [FALSE ("Close Camera") w31] -> w28
                frame False {
                }
                frame True {
                  n360 = call "Display Message to User4"() -> ("Yes"=w32:bool)  [unwired: 10 in, 1 out]
                  n361 = case shown="False" w32 {
                    tunnel: [w33 w34] -> w31
                    frame False {
                      w33 = FALSE ("Close Camera")
                      n362 = local write "Close Camera"(w33) -> ()
                    }
                    frame True {
                      w34 = TRUE ("Close Camera")
                      n363 = local write "Camera Closing"(w34) -> ()
                      n364 = property on="Close Camera" class="Bool (strict)"("DisabledEnum"=T10."Disabled and Grayed Out" ("Disabled")) -> ()  [unwired: 2 in, 2 out]
                    }
                  }
                }
              }
            }
          }
          n365 = Wait (ms)(milliseconds to wait=u32 200) -> ()  [unwired: 1 out]
        }
        n366 = while {
          tunnel: w11 -> [_]
          stop <- w72 stop-if-true
          # "text insertion to .note by control panel"
          n367 = Wait (ms)(milliseconds to wait=u32 200) -> ()  [unwired: 1 out]
          n368 = case shown="True" "Save Note" {
            frame False {
            }
            frame True {
              n369 = flat-sequence {
                frame #0 {
                  n370 = local read "Save"() -> (w75:bool)
                  n371 = case shown="True" w75 {
                    tunnel: [w86 w90] -> w76
                    frame False {
                      n372 = local read "# Saved Fr"() -> (w89:i32)
                      n373 = Number To Decimal String(number=w89) -> (decimal integer string=w88:string)  [unwired: 1 in]
                      n374 = Concatenate Strings(w88, ", last frame") -> (w86:string)
                    }
                    frame True {
                      n375 = local read "# Saved Fr"() -> (w91:i32)
                      n376 = Number To Decimal String(number=w91) -> (decimal integer string=w90:string)  [unwired: 1 in]
                    }
                  }
                  n377 = local read ".note path"() -> (w82:path)
                  n378 = Open/Create/Replace File(file path (use dialog)=w82, operation (0:open)=T11."open or create") -> (refnum out=w83:refnum<file>)  [unwired: 4 in, 2 out]
                  n379 = call ".note text insertion"("frame"=w76, ".notetext"=".note text control") -> ("Result"=w78:string)  [unwired: 12 in, 1 out]
                  n380 = Set File Position(offset (in bytes) (0)=i64 0, refnum=w83, from (0:start)=enum16{"start", "end", "current"}."end") -> (refnum out=w84:refnum<file>)  [unwired: 1 in, 1 out]
                  n381 = Write to Text File(file (use dialog)=w84, text=w78) -> (refnum out=w85:refnum<file>)  [unwired: 2 in, 2 out]
                  n382 = Close File(refnum=w85) -> ()  [unwired: 1 in, 2 out]
                }
                frame #1 {
                  n383 = local write ".note text control"("") -> ()
                }
              }
            }
          }
          n384 = local read "Camera Closing"() -> (w72:bool)
        }
        n385 = stacked-sequence {
          tunnel: w19 -> [w559 _ _ _ _ _ _]
          frame #0 {
            n386 = call "Imaq Dispose"("Image"=w559) -> ()  [unwired: 5 in, 1 out]
            n387 = case shown="False" "Keep cooler on" {
              frame False {
                n388 = call <userlib>:"SetTemperature.vi"("temperature"=20) -> ()  [unwired: 1 in, 2 out]
              }
              frame True {
              }
            }
            n389 = local read "ref image fake"() -> (w557:T4)
            n390 = local write "Live"(FALSE ("Live")) -> ()
            n391 = call <userlib>:"SetShutter.vi"("type"=Shutter_type_typedef."TTL Low", "mode"=Shutter_mode_typedef."Close", "closingtime"=0, "openingtime"=0) -> ()  [unwired: 10 in, 2 out]
            n392 = call "Imaq Dispose"("Image"=w557) -> ()  [unwired: 5 in, 1 out]
          }
          frame #1 {
            n393 = property on="Kill" class="Bool"("Visible"=TRUE) -> ()  [unwired: 2 in, 2 out]
          }
          frame #2 {
            n394 = while {
              stop <- w564 stop-if-true
              n395 = call <userlib>:"GetTemperature.vi"() -> ("temperature"=w567:i32)  [unwired: 4 in, 3 out]
              n396 = Wait (ms)(milliseconds to wait=u32 200) -> ()  [unwired: 1 out]
              n397 = local read "Keep cooler on"() -> (w562:bool)
              n398 = Greater Or Equal?(x=w567, y=0) -> (x >= y?=w565:bool)
              n399 = local write "Temp 2"(w567) -> ()
              n400 = case shown="False" "Kill" {
                tunnel: [w570 TRUE] -> w563
                tunnel: w565 -> [w570 _]
                frame False {
                }
                frame True {
                }
              }
              "Temp>0" <- w563
              n401 = Or(x=w563, y=w562) -> (x .or. y?=w564:bool)
            }
          }
          frame #3 {
            n402 = property on="Kill" class="Bool"("Visible"=FALSE) -> ()  [unwired: 2 in, 2 out]
          }
          frame #4 {
            n403 = local read "Keep cooler on"() -> (w573:bool)
            n404 = case shown="False" w573 {
              frame False {
                n405 = call <userlib>:"CoolerOFF.vi"() -> ()  [unwired: 2 in, 2 out]
              }
              frame True {
              }
            }
            n406 = Wait (ms)(milliseconds to wait=u32 100) -> ()  [unwired: 1 out]
          }
          frame #5 {
            n407 = local read "Keep cooler on"() -> (w575:bool)
            n408 = case shown="False" w575 {
              frame False {
                n409 = call <userlib>:"ShutDown.vi"() -> ()  [unwired: 2 in, 2 out]
              }
              frame True {
              }
            }
          }
          frame #6 {
            w577 = FALSE ("Program Stop")
            w576 = T10."Disabled and Grayed Out" ("Disabled")
            n410 = local write "Start Camera"(w577) -> ()
            n411 = property on="Start Camera" class="Bool (strict)"("DisabledEnum"=T10."Enabled" ("Disabled")) -> ()  [unwired: 2 in, 2 out]
            n412 = local write "Close Camera"(w577) -> ()
            n413 = property on="Rotate" class="Bool (strict)"("DisabledEnum"=w576) -> ()  [unwired: 2 in, 2 out]
            n414 = property on="Reset Scale" class="Bool (strict)"("DisabledEnum"=w576) -> ()  [unwired: 2 in, 2 out]
            n415 = property on="Image 2" class="ImageControl"("DisabledEnum"=w576) -> ()  [unwired: 2 in, 2 out]
            n416 = property on="Zero lower value" class="Bool (strict)"("DisabledEnum"=w576) -> ()  [unwired: 2 in, 2 out]
            n417 = property on="Save Note" class="Bool"("DisabledEnum"=w576) -> ()  [unwired: 2 in, 2 out]
            n418 = property on="Live" class="Bool (strict)"("DisabledEnum"=w576) -> ()  [unwired: 2 in, 2 out]
            n419 = property on="Save" class="Bool (strict)"("DisabledEnum"=w576) -> ()  [unwired: 2 in, 2 out]
            n420 = property on="Previous" class="Bool"("DisabledEnum"=w576) -> ()  [unwired: 2 in, 2 out]
            n421 = property on="Auto Scale" class="Bool (strict)"("DisabledEnum"=w576) -> ()  [unwired: 2 in, 2 out]
            n422 = property on="Image" class="Bool (strict)"("DisabledEnum"=w576) -> ()  [unwired: 2 in, 2 out]
            n423 = property on="Slide" class="Slide (strict)"("DisabledEnum"=w576) -> ()  [unwired: 2 in, 2 out]
          }
        }
      }
    }
    n424 = local read "Stop Program"() -> (w8:bool)
    n425 = local read "Main loop running"() -> (w5:dbl)
    n426 = case shown="True" w8 {
      frame False {
      }
      frame True {
        n427 = local write "Program Closing"(TRUE ("Program Closing")) -> ()
      }
    }
    n428 = local read "Program Closing"() -> (w7:bool)
    n429 = Increment(x=w5) -> (x+1=→"Main loop running":dbl)
    n430 = Wait (ms)(milliseconds to wait=u32 200) -> ()  [unwired: 1 out]
  }
  n431 = flat-sequence {
    tunnel: [TRUE] -> w1
    frame #0 {
      w588 = T10."Disabled and Grayed Out" ("Disabled")
      # "Patternl controls"
      # "General controls"
      n432 = property on="Kill" class="Bool"("Visible"=FALSE) -> ()  [unwired: 2 in, 2 out]
      n433 = property on="Start Camera" class="Bool (strict)"("DisabledEnum"=T10."Enabled" ("Disabled")) -> ()  [unwired: 2 in, 2 out]
      n434 = local write "Stop Program"(FALSE ("Program Stop")) -> ()
      n435 = local write "Start Camera"(FALSE ("Program Stop")) -> ()
      n436 = local write "Close Camera"(FALSE ("Close Camera")) -> ()
      n437 = property on="Slide" class="Slide (strict)"("DisabledEnum"=w588) -> ()  [unwired: 2 in, 2 out]
      n438 = property on="Save Note" class="Bool"("DisabledEnum"=w588) -> ()  [unwired: 2 in, 2 out]
      n439 = property on="Live" class="Bool (strict)"("DisabledEnum"=w588) -> ()  [unwired: 2 in, 2 out]
      n440 = property on="Save" class="Bool (strict)"("DisabledEnum"=w588) -> ()  [unwired: 2 in, 2 out]
      n441 = property on="Reset Scale" class="Bool (strict)"("DisabledEnum"=w588) -> ()  [unwired: 2 in, 2 out]
      n442 = property on="Zero lower value" class="Bool (strict)"("DisabledEnum"=w588) -> ()  [unwired: 2 in, 2 out]
      n443 = property on="Previous" class="Bool"("DisabledEnum"=w588) -> ()  [unwired: 2 in, 2 out]
      n444 = property on="Rotate" class="Bool (strict)"("DisabledEnum"=w588) -> ()  [unwired: 2 in, 2 out]
      n445 = property on="Close Camera" class="Bool (strict)"("DisabledEnum"=w588) -> ()  [unwired: 2 in, 2 out]
      n446 = property on="Auto Scale" class="Bool (strict)"("DisabledEnum"=w588) -> ()  [unwired: 2 in, 2 out]
      n447 = property on="Image" class="Bool (strict)"("DisabledEnum"=w588) -> ()  [unwired: 2 in, 2 out]
      n448 = property on="Image 2" class="ImageControl"("DisabledEnum"=w588) -> ()  [unwired: 2 in, 2 out]
      n449 = local write "Camera starting"(0.0 ("Camera starting")) -> ()
      n450 = local write "Auto Scale"(TRUE ("Auto Scale")) -> ()
      n451 = local write "Rotate"(TRUE ("Rotate")) -> ()
      n452 = property on="Pattern Tab" class="TabCtl (strict)"("Visible"=FALSE) -> ()  [unwired: 2 in, 2 out]
      n453 = property on="Do Stage Jump" class="Bool (strict)"("Value"=FALSE ("Do Stage Jump")) -> ()  [unwired: 2 in, 2 out]
      "Camera Initialized" <- FALSE ("Cam Initialized")
      "Program Closing" <- FALSE ("Program Closing")
      "Camera Closing" <- FALSE ("Camera Closing")
    }
  }
  n454 = while {
    tunnel: w1 -> [_]
    stop <- w605 stop-if-true
    n455 = event shown="[1] \"Analyze Files\": Value Change" {
      selector: _ -> [_ _ _ _ _]
      dyn-events: _ -> [_ _ _ _ _]
      timeout: _ -> [_ _ _ _ _]
      tunnel: [_ _ _ _ w657] -> w603
      event Timeout {
        n456 = event-data() -> ()  [unwired: 1 in, 2 out]
      }
      event "Analyze Files": Value Change {
        n457 = event-data() -> ()  [unwired: 1 in, 5 out]
        n458 = local read "Folder"() -> (w607:path)
        n459 = List Folder(path=w607) -> (folder names=w613:string[])  [unwired: 3 in, 3 out]
        n460 = Array Size(array=w613) -> (size(s)=w612:i32)
        n461 = for {
          N: w612 -> [_]
          tunnel: w613 -> [w614] mode=indexing
          tunnel: w607 -> [w622]
          shift-right: [w617] -> w611
          shift-left: string[] [] -> [w620]
          shift-right: [w616] -> w610
          shift-left: string[] [] -> [w618]
          n462 = Build Path(base path=w622, name or relative path=w614) -> (appended path=w630:path)
          n463 = Concatenate Strings(w614, ".inf" ("pattern")) -> (w633:string)
          n464 = Concatenate Strings(w614, ".dax" ("pattern")) -> (w615:string)
          n465 = Concatenate Strings(w614, ".tif" ("pattern")) -> (w619:string)
          n466 = Build Path(base path=w630, name or relative path=w619) -> (appended path=w627:path)
          n467 = Build Path(base path=w630, name or relative path=w615) -> (appended path=w629:path)
          n468 = Build Path(base path=w630, name or relative path=w633) -> (appended path=w628:path)
          n469 = call <vilib>:"Check if File or Folder Exists.vi"("path"=w629) -> ("file or folder exists?"=w623:bool)  [unwired: 8 in, 2 out]
          n470 = call <vilib>:"Check if File or Folder Exists.vi"("path"=w628) -> ("file or folder exists?"=w624:bool)  [unwired: 8 in, 2 out]
          n471 = call <vilib>:"Check if File or Folder Exists.vi"("path"=w627) -> ("file or folder exists?"=w626:bool)  [unwired: 8 in, 2 out]
          n472 = Not(x=w626) -> (.not. x?=w625:bool)
          n473 = Compound Arithmetic op=AND(w623, w624, w625) -> (w621:bool)
          n474 = case shown="False" w621 {
            tunnel: w620 -> [w638 w642]
            tunnel: w619 -> [w637 _]
            tunnel: w618 -> [w635 w641]
            tunnel: [w636 w642] -> w617
            tunnel: [w635 w640] -> w616
            tunnel: w614 -> [_ w639]
            frame False {
              n475 = Insert Into Array(array=w638, new element=w637) -> (w636:string[])  [unwired: 1 in]
            }
            frame True {
              n476 = Insert Into Array(array=w641, new element=w639) -> (w640:string[])  [unwired: 1 in]
            }
          }
        }
        n477 = local write "List Not Analyzed"(w610) -> ()
        n478 = local write "List Analyzed"(w611) -> ()
      }
      event "Convert Files": Value Change {
        n479 = event-data() -> ()  [unwired: 1 in, 5 out]
        n480 = flat-sequence {
          frame #0 {
            n481 = local read "List Not Analyzed"() -> (w644:string[])
            n482 = local read "List Analyzed"() -> (w647:string[])
            n483 = local read "Folder"() -> (w643:path)
            n484 = Array Size(array=w644) -> (size(s)=w645:i32)
            n485 = for {
              N: w645 -> [_]
              shift-right: [w651] -> w646
              shift-left: w647 -> [w652]
              tunnel: w644 -> [w648] mode=indexing
              tunnel: w643 -> [w649]
              n486 = call "daxinf_to_tif.vi"("String in"=w648, "path in"=w649) -> ()  [unwired: 1 in]
              n487 = Concatenate Strings(w648, ".tif" ("pattern")) -> (w650:string)
              n488 = Insert Into Array(array=w652, new element=w650) -> (w651:string[])  [unwired: 1 in]
            }
            n489 = local write "List Analyzed"(w646) -> ()
          }
          frame #1 {
            n490 = local write "List Not Analyzed"(string[] []) -> ()
          }
        }
      }
      event "Folder": Value Change {
        n491 = event-data() -> ()  [unwired: 1 in, 5 out]
        n492 = local write "List Not Analyzed"(string[] []) -> ()
        n493 = local write "List Analyzed"(string[] []) -> ()
      }
      event "Stop Program": Value Change {
        n494 = event-data() -> ("NewVal"=w657:bool)  [unwired: 1 in, 4 out]
      }
    }
    n495 = Wait (ms)(milliseconds to wait=u32 100) -> ()  [unwired: 1 out]
    n496 = local read "Program Closing"() -> (w606:bool)
    n497 = Or(x=w606, y=w603) -> (x .or. y?=w605:bool)
  }
  n498 = while {
    tunnel: w1 -> [_]
    stop <- w661 stop-if-true
    n499 = event shown="[8] \"Stop Program\": Value Change" {
      selector: _ -> [_ _ _ _ _ _ _ _ _]
      dyn-events: _ -> [_ _ _ _ _ _ _ _ _]
      timeout: _ -> [_ _ _ _ _ _ _ _ _]
      tunnel: [_ _ _ _ _ _ _ _ w689] -> w658
      event Timeout {
        n500 = event-data() -> ()  [unwired: 1 in, 2 out]
      }
      event "ROI 128x128": Value Change {
        n501 = event-data() -> ("NewVal"=w662:bool)  [unwired: 1 in, 4 out]
        n502 = case shown="True" w662 {
          frame False {
          }
          frame True {
            n503 = local write "Hstart"(1 ("hstart")) -> ()
            n504 = local write "Vstart"(1 ("hstart")) -> ()
            n505 = local write "Hend"(128 ("hstart")) -> ()
            n506 = local write "Vend"(128 ("hstart")) -> ()
            n507 = local read "Standard Pixel Size"() -> (w663:bool)
            n508 = case shown="True" w663 {
              frame False {
              }
              frame True {
                n509 = local write "Pixel Size (nm)"(160.0 ("Pixel Size (nm)")) -> ()
              }
            }
            n510 = local write "ROI 512x512"(FALSE ("ROI 512x512")) -> ()
          }
        }
      }
      event "ROI 512x512": Value Change {
        n511 = event-data() -> ("NewVal"=w670:bool)  [unwired: 1 in, 4 out]
        n512 = case shown="True" w670 {
          frame False {
          }
          frame True {
            n513 = local write "Hstart"(1 ("hstart")) -> ()
            n514 = local write "Vstart"(1 ("hstart")) -> ()
            n515 = local write "Hend"(512 ("hstart")) -> ()
            n516 = local write "Vend"(512 ("hstart")) -> ()
            n517 = local read "Standard Pixel Size"() -> (w671:bool)
            n518 = case shown="True" w671 {
              frame False {
              }
              frame True {
                n519 = local write "Pixel Size (nm)"(107.0 ("Pixel Size (nm)")) -> ()
              }
            }
            n520 = local write "ROI 128x128"(FALSE ("ROI 128x128")) -> ()
          }
        }
      }
      event "Hstart": Value Change {
        n521 = event-data() -> ()  [unwired: 1 in, 5 out]
        n522 = local write "ROI 512x512"(FALSE ("ROI 512x512")) -> ()
        n523 = local write "ROI 128x128"(FALSE ("ROI 128x128")) -> ()
      }
      event "Hend": Value Change {
        n524 = event-data() -> ()  [unwired: 1 in, 5 out]
        n525 = local write "ROI 512x512"(FALSE ("ROI 512x512")) -> ()
        n526 = local write "ROI 128x128"(FALSE ("ROI 128x128")) -> ()
      }
      event "Vstart": Value Change {
        n527 = event-data() -> ()  [unwired: 1 in, 5 out]
        n528 = local write "ROI 512x512"(FALSE ("ROI 512x512")) -> ()
        n529 = local write "ROI 128x128"(FALSE ("ROI 128x128")) -> ()
      }
      event "Vend": Value Change {
        n530 = event-data() -> ()  [unwired: 1 in, 5 out]
        n531 = local write "ROI 512x512"(FALSE ("ROI 512x512")) -> ()
        n532 = local write "ROI 128x128"(FALSE ("ROI 128x128")) -> ()
      }
      event "Start Camera": Value Change {
        n533 = event-data() -> ("NewVal"=w686:bool)  [unwired: 1 in, 4 out]
        n534 = case shown="True" w686 {
          frame False {
          }
          frame True {
            n535 = property on="Start Camera" class="Bool (strict)"("DisabledEnum"=T10."Disabled and Grayed Out" ("Disabled")) -> ()  [unwired: 2 in, 2 out]
          }
        }
      }
      event "Stop Program": Value Change {
        n536 = event-data() -> ("NewVal"=w689:bool)  [unwired: 1 in, 4 out]
        n537 = local write "Program Closing"(TRUE ("Program Closing")) -> ()
      }
    }
    n538 = Wait (ms)(milliseconds to wait=u32 100) -> ()  [unwired: 1 out]
    n539 = local read "Program Closing"() -> (w660:bool)
    n540 = Or(x=w660, y=w658) -> (x .or. y?=w661:bool)
  }
  n541 = disable-structure shown="Enabled" {
    disable-tunnel: w1 -> [w691 _]
    frame Enabled {
      n542 = while {
        tunnel: [w705] -> w692
        tunnel: w691 -> [_]
        i -> [w703]
        stop <- w704 continue-if-true
        # "initialize stage"
        n543 = flat-sequence {
          tunnel: [w711] -> w705
          frame #0 {
            n544 = dll-call lib="F:/Vlad/Labview code/PZM_photogate/MCL libraries/MicroDrive.dll" fn="MCL_ReleaseAllHandles"() -> ()  [unwired: 3 in, 3 out]
          }
          frame #1 {
            n545 = dll-call lib="F:/Vlad/Labview code/PZM_photogate/MCL libraries/MicroDrive.dll" fn="MCL_InitHandle" label="MicroDrive.dll:\nMCL_InitHandle"() -> ("handle"=w711:i32)  [unwired: 3 in, 2 out]
          }
        }
        n546 = Equal?(x=w703, y=1) -> (x = y?=w699:bool)
        n547 = case shown="False" w699 {
          tunnel: ["Failed to initialize\na handle for the \nMicroDrive. Retry?" ("message") "Still couldn't initialize a\nhandle for the MicroDrive.\nDevice may not be attaced\nor may be under the control\nof another program. Retry?" ("message")] -> w701
          frame False {
          }
          frame True {
          }
        }
        n548 = Less Or Equal To 0?(x=w705) -> (x <= 0?=w702:bool)
        n549 = case shown="False" w702 {
          tunnel: w701 -> [_ w710]
          tunnel: [FALSE ("T button?") w709] -> w704
          frame False {
          }
          frame True {
            n550 = Two Button Dialog(message=w710) -> (T button?=w709:bool)  [unwired: 2 out]
          }
        }
      }
      n551 = call <vilib>:"Intialize Keyboard.vi"() -> ("device ID"=w697:refnum<k1>)  [unwired: 1 in, 10 out]
      n552 = dll-call lib="F:/Vlad/Labview code/PZM_photogate/MCL libraries/MicroDrive.dll" fn="MCL_MicroDriveCurrentMicroStepPosition"("microStepsX"=0, "microStepsY"=0, "handle"=w692) -> ("handle"=w694:i32)  [unwired: 3 in, 5 out]
      n553 = while {
        tunnel: w694 -> [w716]
        tunnel: [w714] -> w693
        tunnel: w697 -> [w717]
        tunnel: [w717] -> w698
        shift-right: [w712] -> _
        shift-left: "Base Multiplication Factor" -> [w713]
        stop <- w715 stop-if-true
        n554 = stacked-sequence {
          seq-local: [w734 _ _ _] -> [_ w782 _ _]
          seq-local: [w731 _ _ _] -> [_ w784 _ _]
          seq-local: [w722 _ _ _] -> [_ w780 _ _]
          seq-local: [_ w784 _ _] -> [_ _ w850 _]
          seq-local: [_ w783 _ _] -> [_ _ w848 _]
          seq-local: [_ w780 _ _] -> [_ _ w849 _]
          seq-local: [_ _ w842 _] -> [_ _ _ w870]
          tunnel: w717 -> [_ _ _ _]
          tunnel: w716 -> [w737 _ _ _]
          tunnel: w713 -> [w719 _ _ _]
          tunnel: [_ _ w850 _] -> w715
          tunnel: [_ _ _ w871] -> w714
          tunnel: [_ _ w849 _] -> w712
          frame #0 {
            # "8"
            # "4"
            # "2"
            # "1"
            # "RIGHT, LEFT, DOWN, UP"
            # "handle"
            # "axis"
            # "velocity"
            # "move size (um)"
            n555 = call-poly <vilib>:"Acquire Input Data.vi"() -> ("keys pressed"=w758:T5)  [unwired: 2 in, 17 out]
            "keys pressed" <- w758
            n556 = Less?(x="Max Speed Multiplication Factor", y=w719) -> (x < y?=w721:bool)
            n557 = Index Array "Index Array"(array=w758, index=0) -> (element=w743:T17)
            "First Key" <- w743
            n558 = case shown="False" w721 {
              tunnel: "Max Speed Multiplication Factor" -> [_ w761]
              tunnel: w719 -> [w760 _]
              tunnel: [w760 w761] -> w718
              frame False {
              }
              frame True {
              }
            }
            "Current Speed Multiplication factor" <- w718
            n559 = call "InterpretKeyboardCommand.vi"("Key\nValue"=w743, "X Decreasing"="X Decreasing", "X Increasing"="X Increasing", "Y Decreasing"="Y Decreasing", "Y Increasing"="Y Increasing") -> ("number"=w742:u32)  [unwired: 1 in, 5 out]
            n560 = call "ReadKeyboardCommand.vi"("handle"=w737, "Motion #"=w742, "Enable\n(True)"="Gamepad Option") -> ("Enable Move\n(TRUE)"=w730:bool, "Move size (mm)"=w726:dbl, "Axis"=w755:enum16{"X", "Y"})  [unwired: 1 in]
            n561 = Multiply(x="base step size (um)", y=w726) -> (x*y=w724:dbl)
            n562 = Multiply(x=w718, y=w724) -> (x*y=w723:dbl)
            n563 = local read "Program Closing"() -> (w732:bool)
            n564 = local read "Stop Program"() -> (w733:bool)
            n565 = And(x="Gamepad Option", y=w730) -> (x .and. y?=w757:bool)
            n566 = case shown="True" w757 {
              tunnel: w737 -> [w770 w775]
              tunnel: w755 -> [w773 _]
              tunnel: w723 -> [w771 _]
              tunnel: "Velocity (mm/s)" -> [w772 _]
              tunnel: [w764 w775] -> w725
              tunnel: w718 -> [w763 _]
              tunnel: [w762 w774] -> w722
              frame True {
                n567 = To Long Integer(number=w773) -> (32bit integer=w769:i32)
                n568 = Increment(x=w769) -> (x+1=w768:i32)
                n569 = Divide(x=w771, y=1000000.0) -> (x/y=w765:dbl)
                n570 = dll-call lib="F:/Vlad/Labview code/PZM_photogate/MCL libraries/MicroDrive.dll" fn="MCL_MicroDriveMoveProfile" label="MicroDrive.dll:\nMCL_MicroDriveMoveProfile"("axis"=w768, "velocity"=w772, "distance"=w765, "rounding"=0, "handle"=w770) -> ("handle"=w764:i32)  [unwired: 7 in, 3 out]
                n571 = Increment(x=w763) -> (x+1=w762:i32)
              }
              frame False {
                n572 = local read "Base Multiplication Factor"() -> (w774:i32)
              }
            }
            n573 = dll-call lib="F:/Vlad/Labview code/PZM_photogate/MCL libraries/MicroDrive.dll" fn="MCL_MicroDriveCurrentMicroStepPosition"("microStepsX"=0, "microStepsY"=0, "handle"=w725) -> ("handle"=w738:i32)  [unwired: 3 in, 5 out]
            n574 = Or(x=w732, y=w733) -> (x .or. y?=w731:bool)
            n575 = case shown="True" w731 {
              tunnel: w738 -> [w776 w778]
              tunnel: [w776 w777] -> w734
              frame False {
              }
              frame True {
                n576 = dll-call lib="F:/Vlad/Labview code/PZM_photogate/MCL libraries/MicroDrive.dll" fn="MCL_MicroDriveStop" label="MicroDrive.dll:\nMCL_MicroDriveStop"("status"=0, "handle"=w778) -> ("handle"=w777:i32)  [unwired: 3 in, 4 out]
              }
            }
            n577 = Not(x=w730) -> (.not. x?=w729:bool)
            n578 = Wait (ms)(milliseconds to wait=u32 100) -> ()  [unwired: 1 out]
            n579 = call "EncoderRead.vi"("Read Encoder\n= TRUE"=w729, "Reset X"="Reset X", "Reset Y"="Reset Y", "handle"=w734, "Reset  Both"="Reset  Both") -> ("X-Encoder (mm)"=→"X-Encoder (mm)":dbl, "Y-Encoder (mm)"=→"Y-Encoder (mm)":dbl, "X Reverse Limit"=→"X Reverse Limit":bool, "X Forward Limit"=→"X Forward Limit":bool, "Y Reverse Limit"=→"Y Reverse Limit":bool, "Y Forward Limit"=→"Y Forward Limit":bool)
          }
          frame #1 {
            n580 = local read "Do Stage Jump"() -> (w781:bool)
            n581 = case shown="True" w781 {
              tunnel: [w785 w787] -> w783
              tunnel: w782 -> [w785 w788]
              frame False {
              }
              frame True {
                n582 = flat-sequence {
                  tunnel: w788 -> [w790]
                  tunnel: [w790] -> w786
                  tunnel: [w797] -> w787
                  tunnel: w786 -> [w802]
                  frame #0 {
                    n583 = Wait (ms)(milliseconds to wait="Time before stage jump") -> ()  [unwired: 1 out]
                  }
                  frame #1 {
                    w801 = 1 ("roundingX")
                    w800 = 1.5 ("velocityX")
                    w819 = 1000.0 ("y")
                    n584 = To Long Integer(number=enum16{"X", "Y"}."Y" ("Axis 2")) -> (32bit integer=w806:i32)
                    n585 = To Long Integer(number=enum16{"X", "Y"}."X" ("Axis 2")) -> (32bit integer=w807:i32)
                    n586 = Divide(x="Direction to move", y=180.0) -> (x/y=w812:dbl)
                    n587 = Increment(x=w806) -> (x+1=w799:i32)
                    n588 = Increment(x=w807) -> (x+1=w803:i32)
                    n589 = Multiply(x=3.141592653589793, y=w812) -> (x*y=w811:dbl)
                    n590 = Sine & Cosine(0:w811) -> (1:w817:dbl, 2:w816:dbl)
                    n591 = local read "Rotate"() -> (w791:bool)
                    n592 = Multiply(x=w817, y="Jump step\nsize (um)") -> (x*y=w814:dbl)
                    n593 = Multiply(x=w816, y="Jump step\nsize (um)") -> (x*y=w815:dbl)
                    n594 = Divide(x=w814, y=w819) -> (x/y=w794:dbl)
                    n595 = Divide(x=w815, y=w819) -> (x/y=w793:dbl)
                    n596 = flat-sequence {
                      tunnel: w800 -> [w833]
                      tunnel: w795 -> [w832]
                      tunnel: w803 -> [w831]
                      tunnel: w801 -> [w830]
                      tunnel: w802 -> [w829]
                      tunnel: [w828] -> w821
                      tunnel: [w834] -> w820
                      tunnel: w821 -> [w835]
                      tunnel: [w836] -> w798
                      tunnel: w820 -> [w841]
                      tunnel: w801 -> [w840]
                      tunnel: w792 -> [w839]
                      tunnel: w800 -> [w838]
                      tunnel: w799 -> [w837]
                      frame #0 {
                        n597 = dll-call lib="F:/Vlad/Labview code/PZM_photogate/MCL libraries/MicroDrive.dll" fn="MCL_MicroDriveMoveProfile" ("MicroDrive.dll:\nMCL_MicroDriveMoveProfile")("axis"=w831, "velocity"=w833, "distance"=w832, "rounding"=w830, "handle"=w829) -> ("handle"=w828:i32)  [unwired: 7 in, 3 out]
                      }
                      frame #1 {
                        n598 = dll-call lib="F:/Vlad/Labview code/PZM_photogate/MCL libraries/MicroDrive.dll" fn="MCL_MicroDriveWait"("handle"=w835) -> ("handle"=w834:i32)  [unwired: 4 in, 2 out]
                      }
                      frame #2 {
                        n599 = dll-call lib="F:/Vlad/Labview code/PZM_photogate/MCL libraries/MicroDrive.dll" fn="MCL_MicroDriveMoveProfile" ("MicroDrive.dll:\nMCL_MicroDriveMoveProfile")("axis"=w837, "velocity"=w838, "distance"=w839, "rounding"=w840, "handle"=w841) -> ("handle"=w836:i32)  [unwired: 7 in, 3 out]
                      }
                    }
                    n600 = case shown="True" w791 {
                      tunnel: [w823 w824] -> w795
                      tunnel: w794 -> [w823 w825]
                      tunnel: w793 -> [w822 w824]
                      tunnel: [w822 w825] -> w792
                      frame False {
                      }
                      frame True {
                      }
                    }
                    n601 = case shown="False" "Manual Control" {
                      frame False {
                        n602 = flat-sequence {
                          frame #0 {
                            n603 = Wait (ms)(milliseconds to wait="Time before pattern starts") -> ()  [unwired: 1 out]
                          }
                          frame #1 {
                          }
                        }
                      }
                      frame True {
                      }
                    }
                    n604 = disable-structure shown="Disabled" {
                      frame Disabled {
                        n605 = Wait (ms)(milliseconds to wait=u32 200) -> ()  [unwired: 1 out]
                      }
                      frame Enabled {
                      }
                    }
                    n606 = local write "Do Stage Jump"(FALSE ("Do Stage Jump")) -> ()
                    n607 = dll-call lib="F:/Vlad/Labview code/PZM_photogate/MCL libraries/MicroDrive.dll" fn="MCL_MicroDriveWait"("handle"=w798) -> ("handle"=w797:i32)  [unwired: 4 in, 2 out]
                  }
                }
              }
            }
          }
          frame #2 {
            w845 = u32 2 items=["Zoom Tool"=8, "Selection Tool"=0, "Pan Tool"=9, "Point Tool"=1, "Line Tool"=2, "Rectangle Tool"=3, "Rotated Rectangle Tool"=12, "Polyline Tool"=10, "Polygon Tool"=5, "Freehand Tool"=11, "Closed Freehand Tool"=6, "Ellipse Tool"=4, "Annulus Tool"=7] ("Current ROI Tool")
            n608 = property on="Image 2" class="ImageControl"() -> ("Current ROI Tool"=w844:u32)  [unwired: 2 in, 2 out]
            n609 = Equal?(x=w844, y=w845) -> (x = y?=w843:bool)
            n610 = And(x="Move with ROI Line", y=w843) -> (x .and. y?=w846:bool)
            n611 = case shown="True" w846 {
              tunnel: [w851 w853] -> w842
              tunnel: w848 -> [w851 w854]
              frame False {
              }
              frame True {
                n612 = flat-sequence {
                  tunnel: w854 -> [w856]
                  tunnel: [w856] -> w852
                  tunnel: [w861] -> w853
                  tunnel: w852 -> [w862]
                  frame #0 {
                    n613 = local read "Time before stage jump"() -> (w855:u32)
                    n614 = Wait (ms)(milliseconds to wait=w855) -> ()  [unwired: 1 out]
                  }
                  frame #1 {
                    n615 = local read "Rotate"() -> (w860:bool)
                    n616 = property on="Image 2" class="ImageControl"() -> ("ROI"=w858:T9)  [unwired: 2 in, 2 out]
                    n617 = local read "Pixel Size (nm)"() -> (w857:dbl)
                    n618 = call "LineMove.vi"("handle in"=w862, "Rotate"=w860, "ROI"=w858, "Pixel Size (nm)"=w857) -> ("handle out"=w861:i32)  [unwired: 1 in]
                    n619 = local write "Move with ROI Line"(FALSE ("Do Stage Jump")) -> ()
                  }
                }
              }
            }
          }
          frame #3 {
            n620 = case shown="True" "/10" {
              frame False {
              }
              frame True {
                n621 = local read "Step Size (um)"() -> (w877:dbl)
                n622 = Divide(x=w877, y=10.0) -> (x/y=w876:dbl)
                n623 = local write "Step Size (um)"(w876) -> ()
                n624 = local write "/10"(FALSE) -> ()
              }
            }
            n625 = case shown="True" "x10" {
              frame False {
              }
              frame True {
                n626 = local read "Step Size (um)"() -> (w873:dbl)
                n627 = Multiply(x=w873, y=10.0) -> (x*y=w872:dbl)
                n628 = local write "Step Size (um)"(w872) -> ()
                n629 = local write "x10"(FALSE) -> ()
              }
            }
            n630 = Compound Arithmetic op=OR("Left", "Up", "Right", "Down") -> (w865:bool)
            n631 = case shown="True" w865 {
              tunnel: [w880 w883] -> w871
              tunnel: w870 -> [w880 w882]
              frame False {
              }
              frame True {
                n632 = flat-sequence {
                  tunnel: w882 -> [w886]
                  tunnel: [w886] -> w884
                  tunnel: w884 -> [w903]
                  tunnel: [w904] -> w881
                  tunnel: [w937] -> w883
                  tunnel: w881 -> [w937]
                  frame #0 {
                    n633 = local read "Time before stage jump"() -> (w885:u32)
                    n634 = Wait (ms)(milliseconds to wait=w885) -> ()  [unwired: 1 out]
                  }
                  frame #1 {
                    w910 = 1 ("roundingX")
                    w911 = 1.5 ("velocityX")
                    n635 = local read "Down"() -> (w889:bool)
                    n636 = local read "Up"() -> (w890:bool)
                    n637 = local read "Right"() -> (w888:bool)
                    n638 = local read "Left"() -> (w887:bool)
                    n639 = Boolean To (0,1)(Boolean=w890) -> (0, 1=w901:i16)
                    n640 = Boolean To (0,1)(Boolean=w887) -> (0, 1=w898:i16)
                    n641 = Boolean To (0,1)(Boolean=w889) -> (0, 1=w900:i16)
                    n642 = Boolean To (0,1)(Boolean=w888) -> (0, 1=w899:i16)
                    n643 = Divide(x="Step Size (um)", y=1000.0) -> (x/y=w891:dbl)
                    n644 = Subtract(x=w899, y=w898) -> (x-y=w896:i16)
                    n645 = Subtract(x=w901, y=w900) -> (x-y=w897:i16)
                    n646 = To Long Integer(number=enum16{"X", "Y"}."Y" ("Axis 2")) -> (32bit integer=w906:i32)
                    n647 = To Long Integer(number=enum16{"X", "Y"}."X" ("Axis 2")) -> (32bit integer=w905:i32)
                    n648 = Increment(x=w906) -> (x+1=w912:i32)
                    n649 = Increment(x=w905) -> (x+1=w909:i32)
                    n650 = Multiply(x=w891, y=w897) -> (x*y=w895:dbl)
                    n651 = Multiply(x=w891, y=w896) -> (x*y=w894:dbl)
                    n652 = flat-sequence {
                      tunnel: w911 -> [w927]
                      tunnel: w909 -> [w926]
                      tunnel: w910 -> [w925]
                      tunnel: w903 -> [w924]
                      tunnel: [w923] -> w917
                      tunnel: w914 -> [w922]
                      tunnel: [w928] -> w916
                      tunnel: w917 -> [w929]
                      tunnel: [w931] -> w913
                      tunnel: w916 -> [w935]
                      tunnel: w910 -> [w934]
                      tunnel: w911 -> [w933]
                      tunnel: w912 -> [w932]
                      tunnel: w915 -> [w930]
                      frame #0 {
                        n653 = dll-call lib="F:/Vlad/Labview code/PZM_photogate/MCL libraries/MicroDrive.dll" fn="MCL_MicroDriveMoveProfile" ("MicroDrive.dll:\nMCL_MicroDriveMoveProfile")("axis"=w926, "velocity"=w927, "distance"=w922, "rounding"=w925, "handle"=w924) -> ("handle"=w923:i32)  [unwired: 7 in, 3 out]
                      }
                      frame #1 {
                        n654 = dll-call lib="F:/Vlad/Labview code/PZM_photogate/MCL libraries/MicroDrive.dll" fn="MCL_MicroDriveWait"("handle"=w929) -> ("handle"=w928:i32)  [unwired: 4 in, 2 out]
                      }
                      frame #2 {
                        n655 = dll-call lib="F:/Vlad/Labview code/PZM_photogate/MCL libraries/MicroDrive.dll" fn="MCL_MicroDriveMoveProfile" ("MicroDrive.dll:\nMCL_MicroDriveMoveProfile")("axis"=w932, "velocity"=w933, "distance"=w930, "rounding"=w934, "handle"=w935) -> ("handle"=w931:i32)  [unwired: 7 in, 3 out]
                      }
                    }
                    n656 = local read "Rotate"() -> (w902:bool)
                    n657 = case shown="True" w902 {
                      tunnel: w895 -> [w919 w920]
                      tunnel: [w919 w921] -> w914
                      tunnel: [w918 w920] -> w915
                      tunnel: w894 -> [w918 w921]
                      frame False {
                      }
                      frame True {
                      }
                    }
                    n658 = dll-call lib="F:/Vlad/Labview code/PZM_photogate/MCL libraries/MicroDrive.dll" fn="MCL_MicroDriveWait"("handle"=w913) -> ("handle"=w904:i32)  [unwired: 4 in, 2 out]
                  }
                  frame #2 {
                    w936 = FALSE
                    n659 = local write "Down"(w936) -> ()
                    n660 = local write "Right"(w936) -> ()
                    n661 = local write "Left"(w936) -> ()
                    n662 = local write "Up"(w936) -> ()
                  }
                }
              }
            }
          }
        }
      }
      n663 = call-poly <vilib>:"Close Input Device.vi"("device ID"=w698) -> ()  [unwired: 1 in, 9 out]
      n664 = dll-call lib="F:/Vlad/Labview code/PZM_photogate/MCL libraries/MicroDrive.dll" fn="MCL_ReleaseHandle" label="MicroDrive.dll:\nMCL_ReleaseHandle"("handle"=w693) -> ()  [unwired: 4 in, 3 out]
    }
    frame Disabled {
    }
  }
  n665 = disable-structure shown="Enabled" {
    disable-tunnel: w1 -> [w939 _]
    frame Enabled {
      n666 = while {
        tunnel: w939 -> [_]
        tunnel: [FALSE ("Stop Program")] -> w938
        stop <- w944 stop-if-true
        # "Shutters and piezo mirror control"
        n667 = flat-sequence {
          tunnel: [w954] -> w942
          tunnel: [w952] -> w941
          tunnel: [w947] -> w940
          tunnel: w942 -> [w1067]
          tunnel: w941 -> [w1066]
          tunnel: w940 -> [w1065]
          frame #0 {
            w950 = 0 items=["one channel for each line", "one channel for all lines"] ("line grouping")
            w963 = 10348 items=["Volts"=10348, "From Custom Scale"=10065] ("units")
            n668 = call-poly <vilib>:"DAQmx Create Virtual Channel.vi"("maximum value"=10.0, "minimum value"=0.0, "physical channels"=tag "Dev1/ao0:1", "units"=w963) -> ("task out"=w962:refnum<k21>, "error out"=w961:errorcluster)  [unwired: 10 in]
            n669 = Build Array("Piezo mirror X (V)", "Piezo mirror Y (V)") -> (w958:dbl[])
            n670 = call-poly <vilib>:"DAQmx Create Virtual Channel.vi"("lines"=tag "Dev1/port0/line0", "line grouping"=w950) -> ("task out"=w948:refnum<k21>, "error out"=w949:errorcluster)  [unwired: 12 in]
            n671 = case shown="\"Spiral to circle\"" "Control type" {
              tunnel: w962 -> [w987 w1009 w1013]
              tunnel: w961 -> [w986 w1008 w1020]
              tunnel: w958 -> [w977 _ _]
              tunnel: "Mirror pattern params" -> [_ w997 w1019]
              tunnel: [w974 w990 w1035] -> w952
              tunnel: [w968 w989 w1024] -> w954
              tunnel: "Photogate" -> [w968 w989 w1023]
              tunnel: "Shutter control" -> [_ _ w1025]
              tunnel: w949 -> [_ _ w1030]
              tunnel: w948 -> [_ _ w1028]
              tunnel: [sgl 0.0 ("Actual Expsoure") sgl 0.0 ("Actual Expsoure") "Imaging delay (ms)"] -> w947
              frame "Manual Control", Default {
                w970 = -5.0 ("x")
                n672 = call-poly <vilib>:"DAQmx Write.vi"("task/channels in"=w987, "data"=w977, "error in"=w986) -> ("task out"=w983:refnum<k21>, "error out"=w981:errorcluster)  [unwired: 10 in, 1 out]
                n673 = Index Array(array=w977, index=1) -> (element=w972:dbl)
                n674 = Index Array(array=w977, index=0) -> (element=w969:dbl)
                n675 = Add(x=w969, y=w970) -> (x+y=w973:dbl)
                n676 = Add(x=w970, y=w972) -> (x+y=w971:dbl)
                n677 = call <vilib>:"DAQmx Start Task.vi"("task/channels in"=w983, "error in"=w981) -> ("task out"=w982:refnum<k21>, "error out"=w985:errorcluster)  [unwired: 12 in]
                n678 = Build Array(w973) -> (w976:dbl[])
                n679 = call <vilib>:"DAQmx Clear Task.vi"("task in"=w982, "error in"=w985) -> ("error out"=w984:errorcluster)  [unwired: 13 in]
                n680 = Build Array(w971) -> (w975:dbl[])
                n681 = call <vilib>:"General Error Handler.vi"("error in (no error)"=w984) -> ()  [unwired: 10 in, 5 out]
                n682 = Bundle(w976, w975) -> (w974:cluster{dbl[], dbl[]})  [unwired: 1 in]
                n683 = Wait (ms)(milliseconds to wait=u32 50) -> ()  [unwired: 1 out]
              }
              frame "Single pattern" {
                n684 = Unbundle By Name(w997) -> ("Start radius (V)"=w994:dbl, "End radius (V)"=w993:dbl, "Ring duration (s)"=w996:dbl, "Mirror loop rate (Hz)"=w995:dbl)
                n685 = Multiply(x=w996, y=w995) -> (x*y=w991:dbl)
                n686 = call-poly <vilib>:"DAQmx Timing.vi"("task/channels in"=w1009, "samples per channel"=w991, "rate"=w995, "error in"=w1008) -> ("task out"=w1007:refnum<k21>, "error out"=w1006:errorcluster)  [unwired: 10 in]
                n687 = call "GenerateSpiralOrCircle.vi"("Number of elements"=w991, "End radius (V)"=w993, "Start radius (V)"=w994) -> ("2D array to piezo mirror"=w992:dbl[][], "Output pattern (cluster)"=w990:cluster{dbl[], dbl[]})  [unwired: 1 in]
                n688 = call-poly <vilib>:"DAQmx Write.vi"("task/channels in"=w1007, "auto start"=FALSE, "data"=w992, "error in"=w1006) -> ("task out"=w1005:refnum<k21>, "error out"=w1004:errorcluster)  [unwired: 9 in, 1 out]
                n689 = call <vilib>:"DAQmx Start Task.vi"("task/channels in"=w1005, "error in"=w1004) -> ("task out"=w1002:refnum<k21>, "error out"=w1001:errorcluster)  [unwired: 12 in]
                n690 = call <vilib>:"DAQmx Wait Until Done.vi"("task/channels in"=w1002, "error in"=w1001) -> ("task out"=w999:refnum<k21>, "error out"=w998:errorcluster)  [unwired: 12 in]
                n691 = call <vilib>:"DAQmx Clear Task.vi"("task in"=w999, "error in"=w998) -> ("error out"=w1000:errorcluster)  [unwired: 13 in]
                n692 = call <vilib>:"General Error Handler.vi"("error in (no error)"=w1000) -> ()  [unwired: 10 in, 5 out]
              }
              frame "Spiral to circle" {
                n693 = Unbundle By Name(w1019) -> ("Number of spirals"=w1033:u32, "Start radius (V)"=w1011:dbl, "End radius (V)"=w1034:dbl, "Time between \ngates (ms)"=w1010:u32)
                n694 = Unbundle By Name(w1019) -> ("Ring duration (s)"=w1037:dbl, "Mirror loop rate (Hz)"=w1036:dbl)
                n695 = Multiply(x=w1037, y=w1036) -> (x*y=w1017:dbl)
                n696 = call "Calculate spiral radii for current iteration.vi"("Number of spirals"=w1033, "Start radius (V)"=w1011, "End radius (V)"=w1034, "Run pattern"="Run pattern", "Time between post-bleaching\ngates (ms)"=w1010) -> ("Radius 1"=w1032:dbl, "Radius 2"=w1031:dbl)  [unwired: 1 in, 1 out]
                n697 = Merge Errors(w1020, w1030) -> (w1012:errorcluster)
                n698 = call "GenerateSpiralOrCircle.vi"("Number of elements"=w1017, "Pattern running?"="Run pattern", "End radius (V)"=w1031, "Start radius (V)"=w1032) -> ("2D array to piezo mirror"=w1016:dbl[][], "Output pattern (cluster)"=w1035:cluster{dbl[], dbl[]})
                n699 = Select(t="Run pattern", s=w1025, f=w1023) -> (s? t:f=w1027:bool)
                n700 = flat-sequence {
                  tunnel: [w1050] -> w1029
                  tunnel: w1028 -> [w1049]
                  tunnel: w1027 -> [w1048]
                  tunnel: [w1040] -> w1021
                  tunnel: w1019 -> [w1045]
                  tunnel: [w1044] -> w1018
                  tunnel: w1016 -> [w1041]
                  tunnel: [w1038] -> w1015
                  tunnel: w1013 -> [w1040]
                  tunnel: w1012 -> [w1039]
                  tunnel: w1029 -> [w1057]
                  tunnel: w1016 -> [w1060]
                  tunnel: w1021 -> [w1055]
                  tunnel: w1018 -> [w1053]
                  tunnel: w1015 -> [w1052]
                  frame #0 {
                    n701 = Unbundle By Name(w1045) -> ("Mirror loop rate (Hz)"=w1044:dbl)
                    n702 = call-poly <vilib>:"DAQmx Write.vi"("task/channels in"=w1049, "auto start"=TRUE, "data"=w1048, "error in"=w1039) -> ("task out"=w1046:refnum<k21>, "error out"=w1047:errorcluster)  [unwired: 9 in, 1 out]
                    n703 = Array Size(array=w1041) -> (size(s)=w1042:i32[])
                    n704 = call <vilib>:"DAQmx Clear Task.vi"("task in"=w1046, "error in"=w1047) -> ("error out"=w1050:errorcluster)  [unwired: 13 in]
                    n705 = Index Array(array=w1042, index=1) -> (element=w1038:i32)
                  }
                  frame #1 {
                    n706 = call-poly <vilib>:"DAQmx Timing.vi"("task/channels in"=w1055, "samples per channel"=w1052, "rate"=w1053, "error in"=w1057) -> ("task out"=w1054:refnum<k21>, "error out"=w1056:errorcluster)  [unwired: 10 in]
                    n707 = call-poly <vilib>:"DAQmx Write.vi"("task/channels in"=w1054, "auto start"=TRUE, "data"=w1060, "error in"=w1056) -> ("task out"=w1061:refnum<k21>, "error out"=w1059:errorcluster)  [unwired: 9 in, 1 out]
                    n708 = call <vilib>:"DAQmx Wait Until Done.vi"("task/channels in"=w1061, "error in"=w1059) -> ("task out"=w1063:refnum<k21>, "error out"=w1064:errorcluster)  [unwired: 12 in]
                    n709 = call <vilib>:"DAQmx Clear Task.vi"("task in"=w1063, "error in"=w1064) -> ("error out"=w1062:errorcluster)  [unwired: 13 in]
                    n710 = call <vilib>:"General Error Handler.vi"("error in (no error)"=w1062) -> ()  [unwired: 10 in, 5 out]
                  }
                }
                n711 = Select(t=FALSE, s=w1025, f=w1023) -> (s? t:f=w1024:bool)
              }
            }
          }
          frame #1 {
            w1081 = 0 items=["one channel for each line", "one channel for all lines"] ("line grouping")
            n712 = Tick Count (ms)() -> (millisecond timer value=w1069:u32)
            n713 = feedback #6() -> (w1070:u32)  [unwired: 1 in]
            n714 = Subtract(x=w1069, y=w1070) -> (x-y=w1071:u32)
            n715 = feedback-in #6(w1069) -> ()
            n716 = Divide(x=w1071, y=u32 1000) -> (x/y=→"Piezo mirror\nloop duration (s)":dbl)
            n717 = call-poly <vilib>:"DAQmx Create Virtual Channel.vi"("lines"=tag "Dev1/port0/line0", "line grouping"=w1081) -> ("task out"=w1079:refnum<k21>, "error out"=w1078:errorcluster)  [unwired: 12 in]
            n718 = Wait (ms)(milliseconds to wait=w1065) -> ()  [unwired: 1 out]
            n719 = call-poly <vilib>:"DAQmx Write.vi"("task/channels in"=w1079, "data"=w1067, "error in"=w1078) -> ("task out"=w1077:refnum<k21>, "error out"=w1076:errorcluster)  [unwired: 10 in, 1 out]
            n720 = call <vilib>:"DAQmx Start Task.vi"("task/channels in"=w1077, "error in"=w1076) -> ("task out"=w1075:refnum<k21>, "error out"=w1074:errorcluster)  [unwired: 12 in]
            n721 = call <vilib>:"DAQmx Clear Task.vi"("task in"=w1075, "error in"=w1074) -> ("error out"=w1073:errorcluster)  [unwired: 13 in]
            n722 = call <vilib>:"General Error Handler.vi"("error in (no error)"=w1073) -> ()  [unwired: 10 in, 5 out]
            "Piezo mirror position" <- w1066
          }
        }
        n723 = local read "Program Closing"() -> (w946:bool)
        n724 = local read "Stop Program"() -> (w945:bool)
        n725 = Or(x=w946, y=w945) -> (x .or. y?=w944:bool)
      }
      n726 = local write "Stop Program"(w938) -> ()
    }
    frame Disabled {
    }
  }
  n727 = local write "Main loop running"(w2) -> ()
